vi "Interpolate_Calib_Coeff.vi"(5 "Analysis Info cluster":T1={"Colour"=0, "Inst type"=enum."Pitot-static tube", "Inst name"="Manometer voltage", "Symbol"="U", "Code name"="", "Extra Info"="U", "Inst Array"=enum."PWA", "U"=0.0, "u^2"=0.0, "u^3"=0.0, "u^4"=0.0, "Skew_u"=0.0, "Kurt_u"=0.0, "Sd Error in Mean"=0.0, "% u'/U"=0.0, "X"=0.0, "Y"=0.0, "Z"=0.0, "Timescale integral Estimate"=0.0, "Sd Error in Variance"=0.0, "Calib File"=path "", "Calib Constants"=[], "Output Position"=FALSE, "Stats"=enum."None", "Av Sampling Rate"=0.0, "Av No of Samples"=0.0, "Total Meas Time (s)"=0.0, "OrigChName"="", "Max value"=0.0, "Min value"=0.0, "Req Sample Rate Hz"=0.0, "Sync Delay Time (s)"=0.0, "Ch No"=0, "Device"="", "Use Latest Calib"=FALSE, "Port"="", "Metadata Ch Names"=[], "Metadata Ch Values"=[], "Label"="", "chState"=enum."Solo", "Point Drift"=0.0, "inputConfig"=""} {"Kurt_u" format="%_3g"; "u^4" format="%_3g"; "u^3" format="%_3g"; "Sd Error in Variance" format="%_3g"; "u^2" format="%_3g"; "Sd Error in Mean" format="%_3g"; "U" format="%_3g"; "Sync Delay Time (s)" format="%.4f"; "Total Meas Time (s)" format="%_5g"; "Skew_u" format="%_3g"; "% u'/U" format="%_3g"}, 7 "Take New Data?":bool) -> (0 "Calib Coeff":dbl[](array[numeric]), 1 "Calib Type Name":string, 2 "Calib file string":string, 3 "Read file":bool, 4 "Analysis Info cluster  Out":T1={"Colour"=0, "Inst type"=enum."Pitot-static tube", "Inst name"="Manometer voltage", "Symbol"="U", "Code name"="", "Extra Info"="U", "Inst Array"=enum."PWA", "U"=0.0, "u^2"=0.0, "u^3"=0.0, "u^4"=0.0, "Skew_u"=0.0, "Kurt_u"=0.0, "Sd Error in Mean"=0.0, "% u'/U"=0.0, "X"=0.0, "Y"=0.0, "Z"=0.0, "Timescale integral Estimate"=0.0, "Sd Error in Variance"=0.0, "Calib File"=path "", "Calib Constants"=[], "Output Position"=FALSE, "Stats"=enum."None", "Av Sampling Rate"=0.0, "Av No of Samples"=0.0, "Total Meas Time (s)"=0.0, "OrigChName"="", "Max value"=0.0, "Min value"=0.0, "Req Sample Rate Hz"=0.0, "Sync Delay Time (s)"=0.0, "Ch No"=0, "Device"="", "Use Latest Calib"=FALSE, "Port"="", "Metadata Ch Names"=[], "Metadata Ch Values"=[], "Label"="", "chState"=enum."Solo", "Point Drift"=0.0, "inputConfig"=""} {"Kurt_u" format="%_3g"; "u^4" format="%_3g"; "u^3" format="%_3g"; "Sd Error in Variance" format="%_3g"; "u^2" format="%_3g"; "Sd Error in Mean" format="%_3g"; "U" format="%_3g"; "Sync Delay Time (s)" format="%.4f"; "Total Meas Time (s)" format="%_5g"; "Skew_u" format="%_3g"; "% u'/U" format="%_3g"})   [LabVIEW 2022 SP3]
uses:
  Controls/Inst_type.ctl
  Globals/Meas_global.vi
  <vilib>/Analysis/NI_AALPro.lvlib
  Globals/Plug_in_data_global.vi
  XW calib map/XW_Map_Global.vi
  XW calib map/Map method.ctl
  Globals/Dynamic_call_global.ph.vi
  <vilib>/Analysis/NI_AALBase.lvlib
  <vilib>/Analysis/baseanly.llb/Mean (DBL).vi
  FFID/FFID Calib Constants index.ctl
  CTA/CTA Calib Coeff Global.vi
  Controls/Analysis_info_cluster.ctl
  Controls/Instrument_Array.ctl
  Controls/channelState.ctl
panel:
  out "Volts":dbl
  out "Time":dbl format="%#.0f"
  out "Earlier raw data file":string
  in  "TAKE NEW DATA XW Map method":T5=enum."Const. Psi_eff (std.)"
  in  "Domain padding factor":dbl=1.01
  in  "cap indicial sum to n":bool=TRUE
  in  "surface order (n)":i32=5
  in  "Apply calibration corrections":bool=TRUE
  in  "POST PROC. XW Map method":T5=enum."Psi_eff, k = f(Umagn.)"
  in  "variable n":bool=TRUE
  in  "wire diameter (mu.m)":dbl=5.0
  out "Header info":string[][](array[string])
  # "For polysurface method only:"
  # "For trimesh method only"
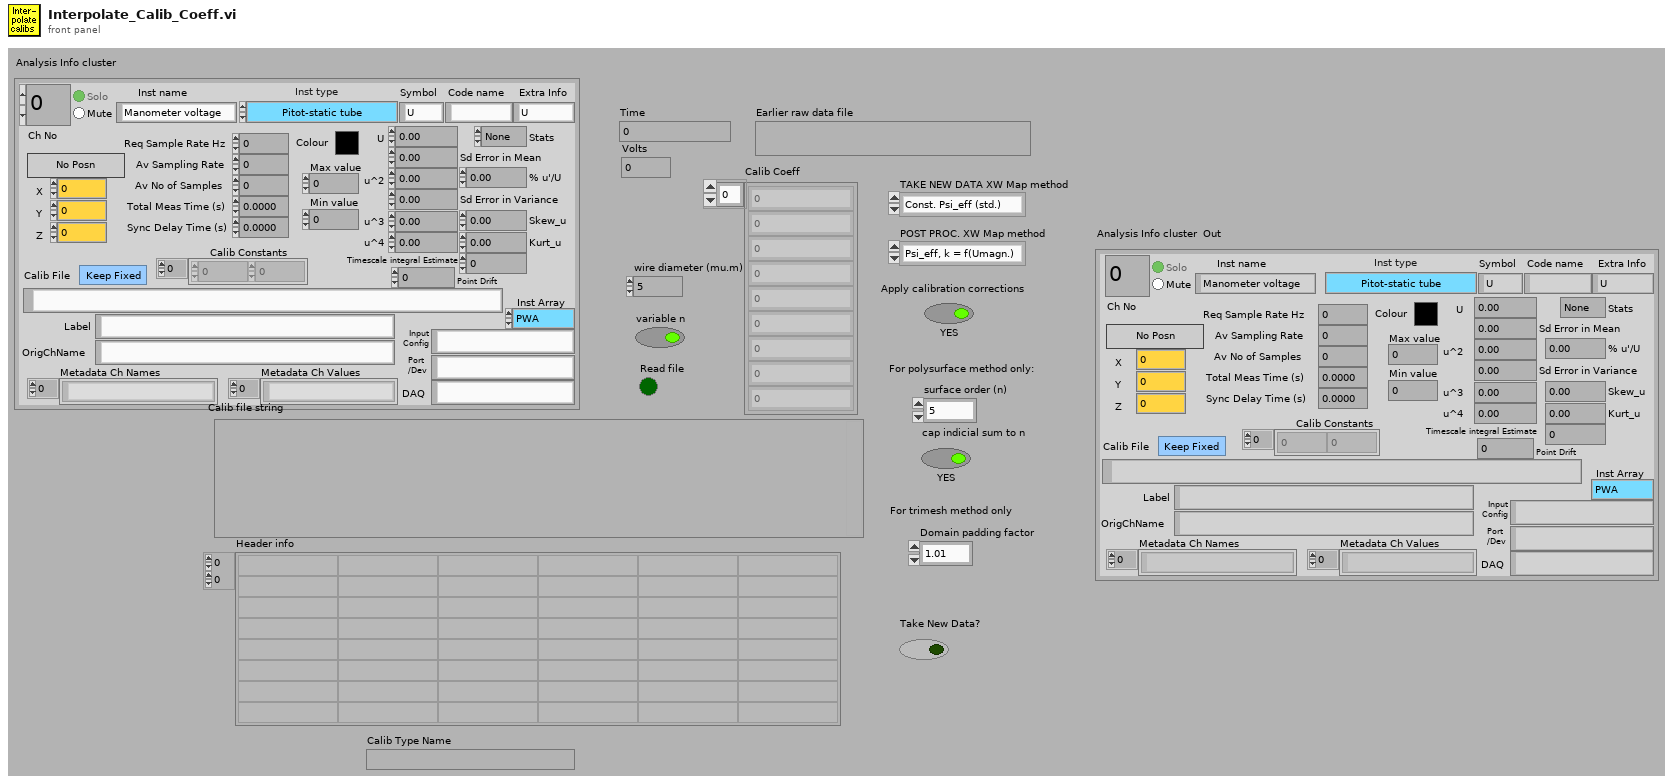
[diagram p1: front panel]
types:
  T1 = typedef "Analysis_info_cluster.ctl" = cluster{"Colour":u32, "Inst type":T2, "Inst name":string, "Symbol":string, "Code name":string, "Extra Info":string, "Inst Array":T3, "U":dbl, "u^2":dbl, "u^3":dbl, "u^4":dbl, "Skew_u":dbl, "Kurt_u":dbl, "Sd Error in Mean":dbl, "% u'/U":dbl, "X":dbl, "Y":dbl, "Z":dbl, "Timescale integral Estimate":dbl, "Sd Error in Variance":dbl, "Calib File":path, "Calib Constants":dbl[], "Output Position":bool, "Stats":enum16{"None", "Basic", "Full"}, "Av Sampling Rate":dbl, "Av No of Samples":dbl, "Total Meas Time (s)":dbl, "OrigChName":string, "Max value":dbl, "Min value":dbl, "Req Sample Rate Hz":dbl, "Sync Delay Time (s)":dbl, "Ch No":i16, "Device":string, "Use Latest Calib":bool, "Port":string, "Metadata Ch Names":string[], "Metadata Ch Values":string[], "Label":string, "chState":T4, "Point Drift":dbl, "inputConfig":string}
  T2 = typedef "Inst_type.ctl" = enum16{"Raw voltage", "Raw with zero offsetting", "Propeller anemometer", "Pressure Transducer", "Pitot-static tube", "Hot wire", "Cross wire 1", "Cross wire 2", "Generic Linear", "Generic Polynomial", "Generic BackPoly", "Fast FID", "Thermocouple", "Cold wire", "Pulsed Wire", "LDA Vel", "LDA Tran time", "LDA Arr time", "Microphone"}
  T3 = typedef "Instrument_Array.ctl" = enum16{"PWA", "LDA", "Analogue"}
  T4 = typedef "channelState.ctl" = enum32{"No Selection", "Solo", "Mute"}
  T5 = typedef "Map method.ctl" = enum16{"Triangle mesh", "Polynomial surface", "Const. Psi_eff (std.)", "Psi_eff = f(Umagn.)", "Psi_eff, k = f(Umagn.)"}
  T6 = cluster{"1st Calib time":dbl, "2nd Calib time":dbl, "Meas start time":dbl, "Meas end time":dbl, "Fraction":dbl}
  T7 = enum16{"Save no data", "Save data in new files", "Save data in existing files"}
  T8 = typedef "Calibration data.ctl" = cluster{"X cal.[]":dbl[], "Re cal.[]":dbl[], "a1[]":dbl[], "a2[]":dbl[], "a3[]":dbl[]}
  T9 = typedef "FFID Calib Constants index.ctl" = u16
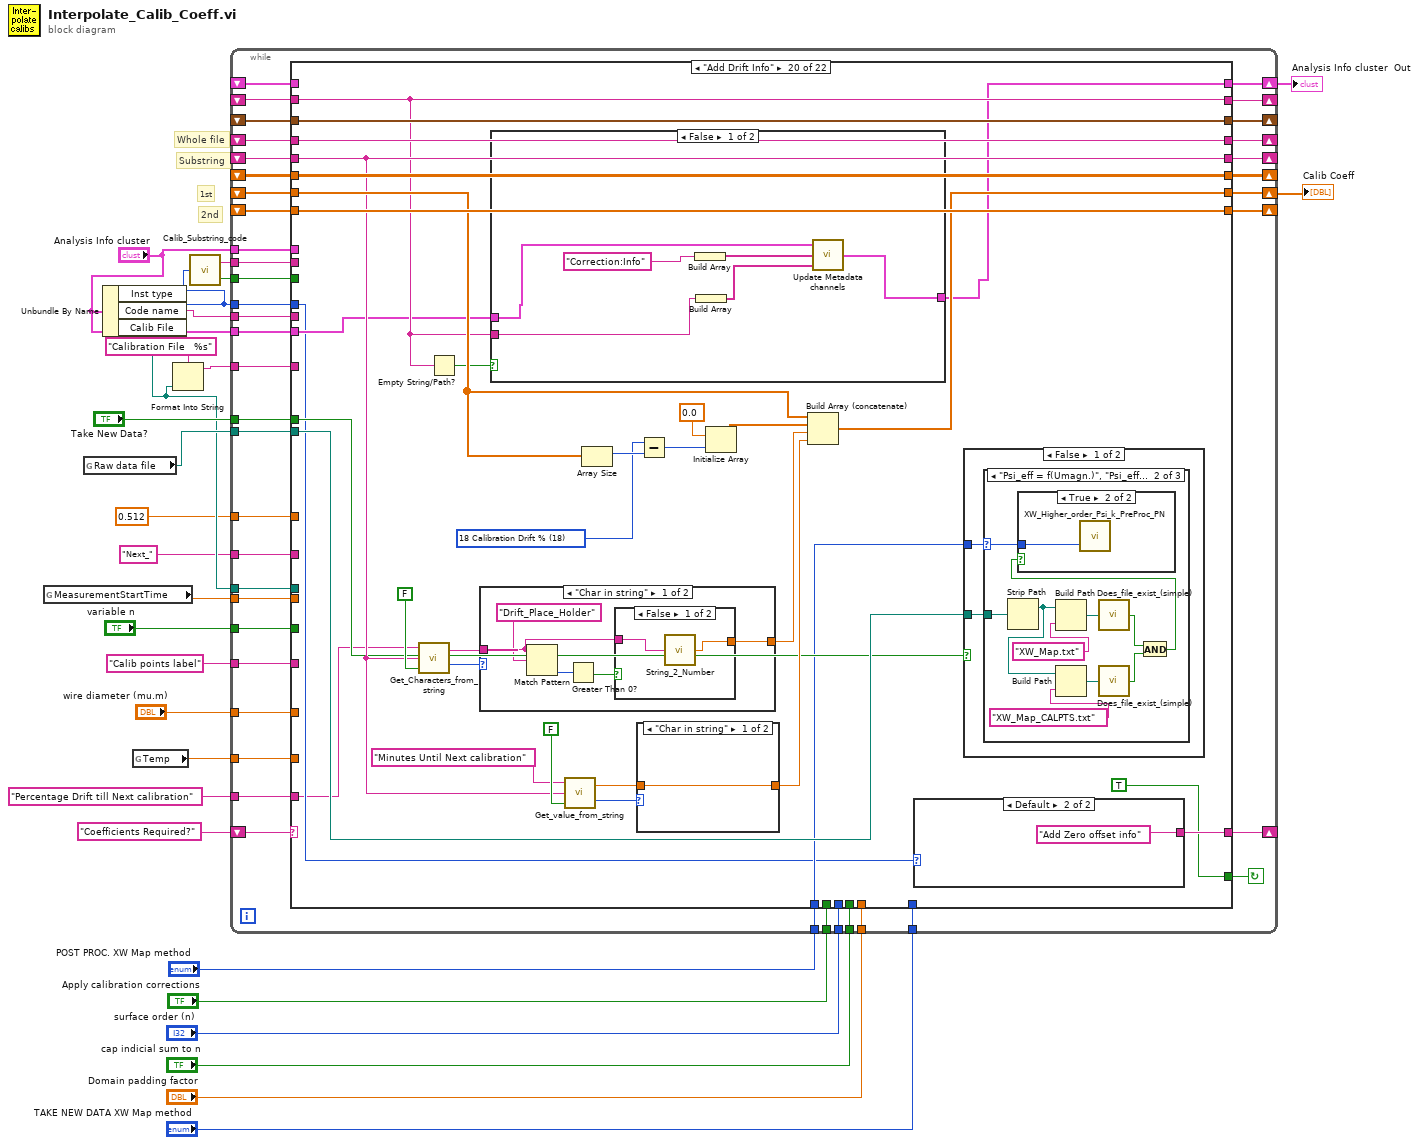
[diagram p0: block diagram]
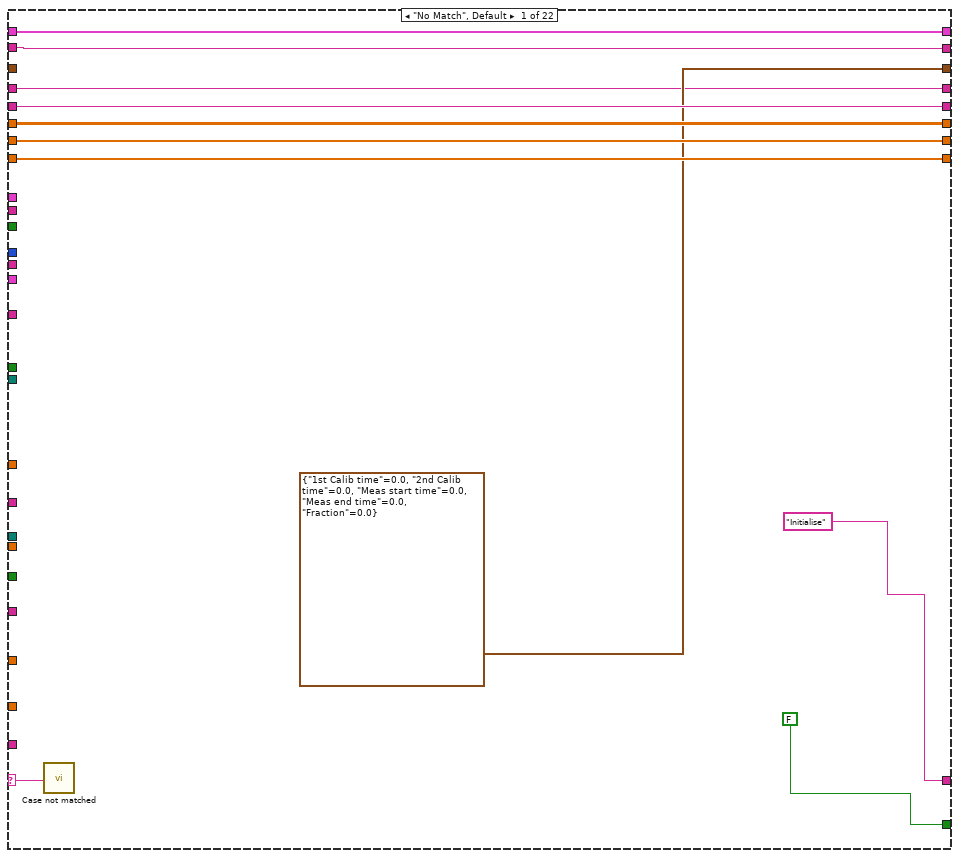
[diagram p2: hidden frame]
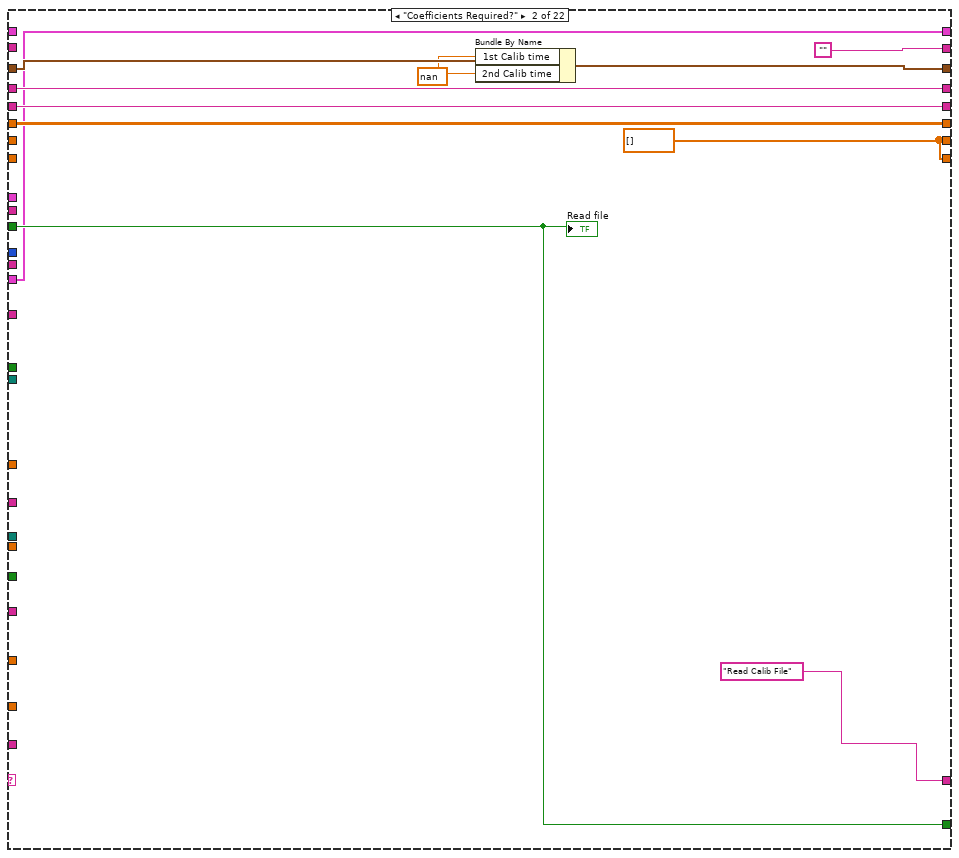
[diagram p3: hidden frame]
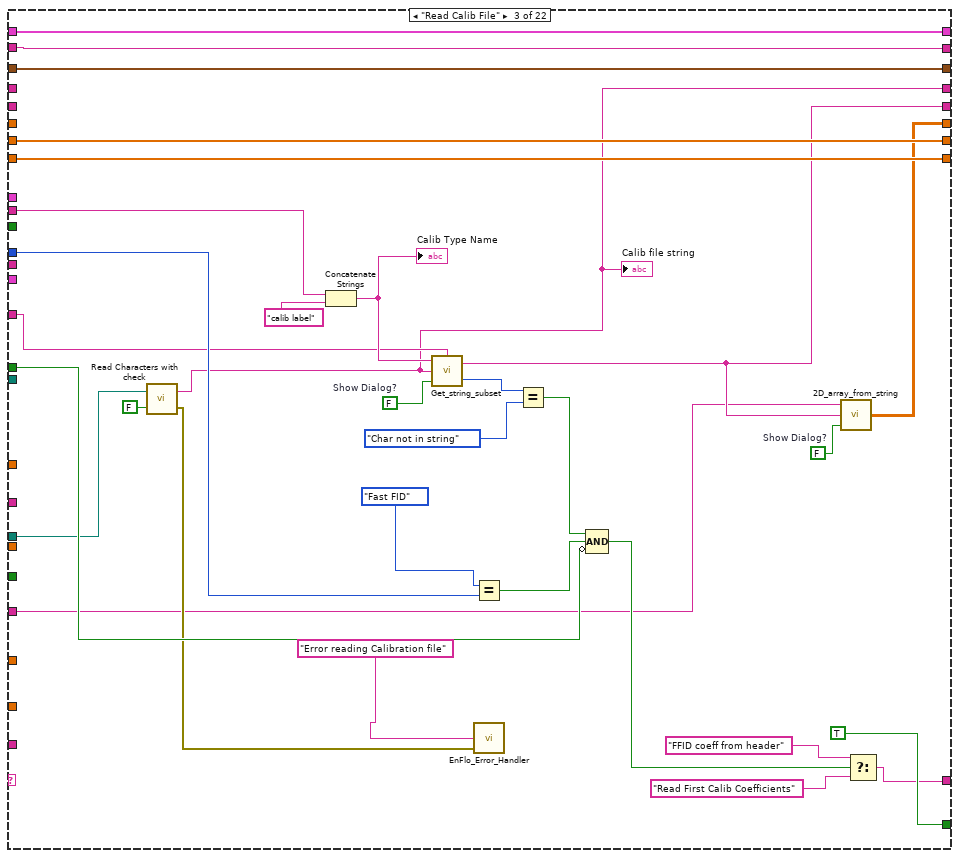
[diagram p4: hidden frame]
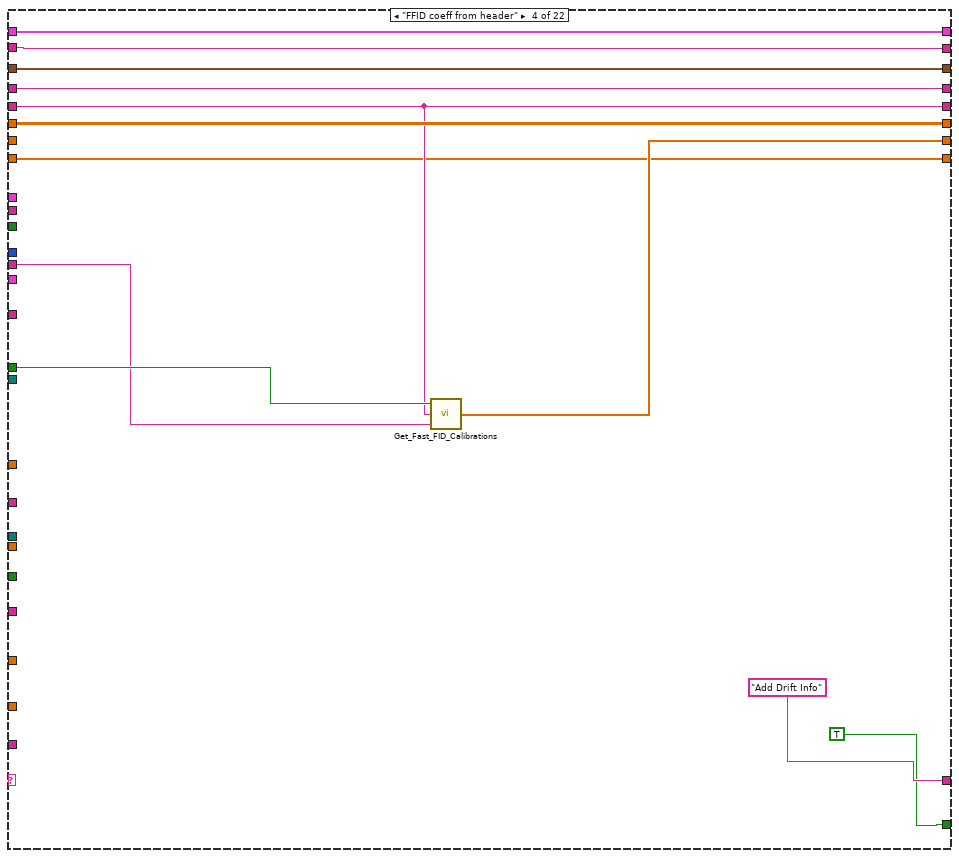
[diagram p5: hidden frame]
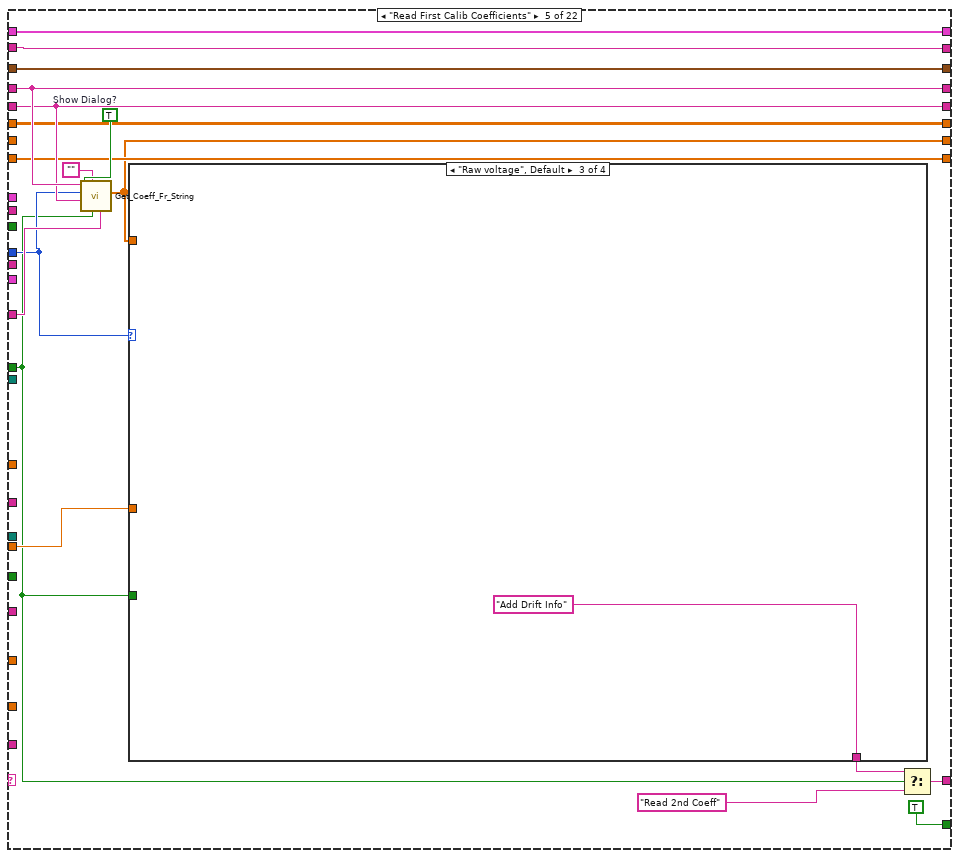
[diagram p6: hidden frame]
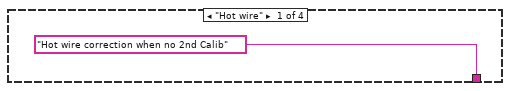
[diagram p7: hidden frame]
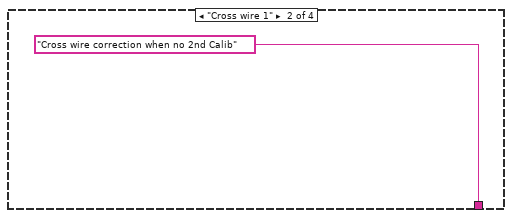
[diagram p8: hidden frame]
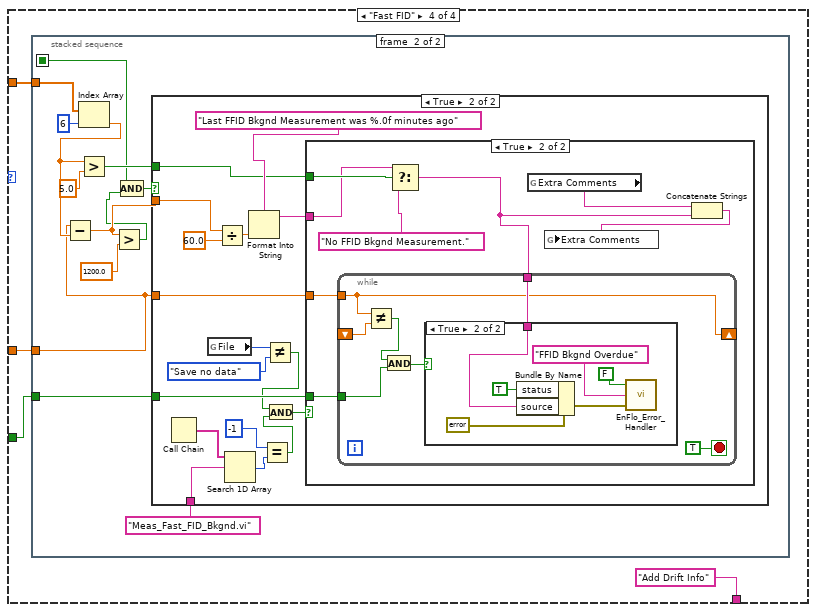
[diagram p9: hidden frame]
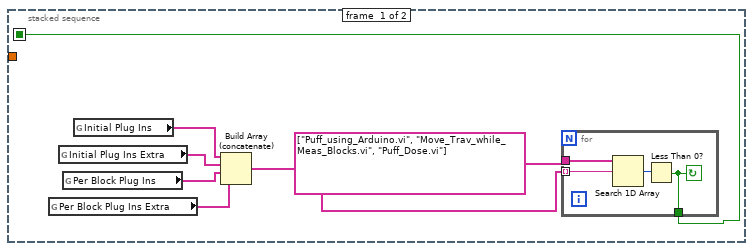
[diagram p10: hidden frame]
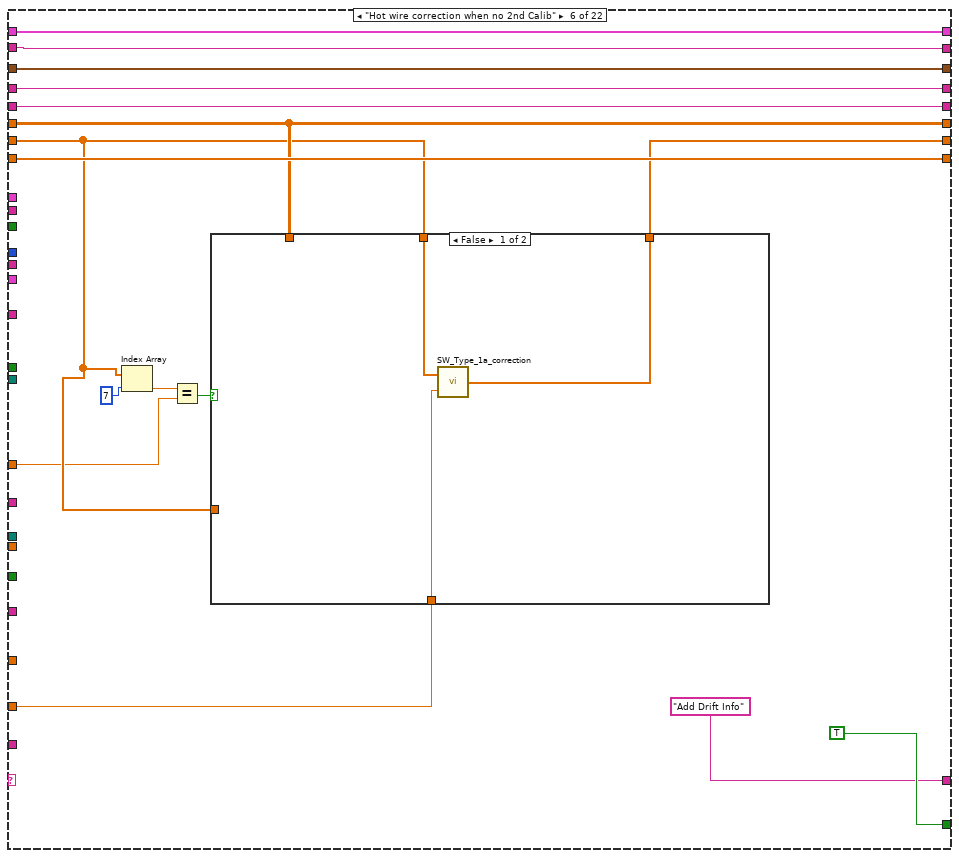
[diagram p14: hidden frame]
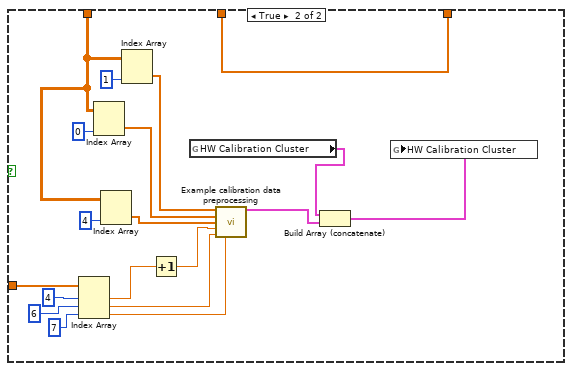
[diagram p15: hidden frame]
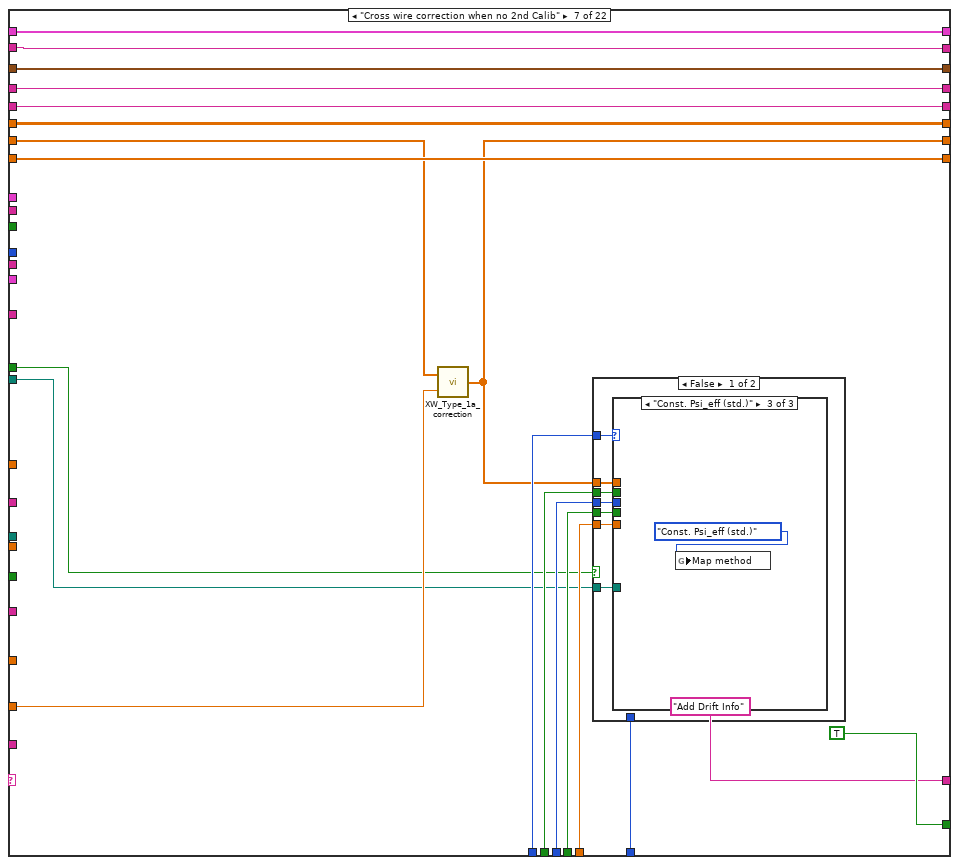
[diagram p16: hidden frame]
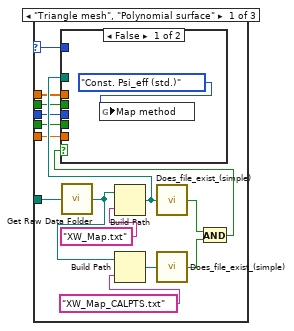
[diagram p17: hidden frame]
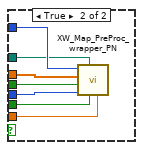
[diagram p18: hidden frame]
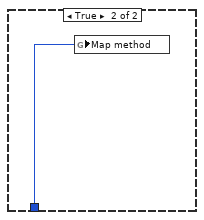
[diagram p20: hidden frame]
diagram:
  # "Substring"
  # "2nd"
  # "Whole file"
  # "1st"
  n1 = global read "Meas_global.vi" "MeasurementStartTime"() -> (w5:dbl)
  n2 = global read "Meas_global.vi" "Raw data file"() -> (w21:path)
  n3 = Unbundle By Name("Analysis Info cluster") -> ("Inst type"=w24:T2, "Code name"=w25:string, "Calib File"=w7:path)
  n4 = global read "Meas_global.vi" "Temp"() -> (w20:dbl)
  n5 = Format Into String(format string="Calibration File   %s", w7) -> (resulting string=w8:string)  [unwired: 2 in, 1 out]
  n6 = call "Calib_Substring_code.vi"("Inst type"=w24) -> ("Substring Type"=w22:string, "Read file"=w23:bool)
  n7 = while {
    tunnel: w7 -> [w61]
    shift-left: _ -> [w62]
    shift-right: [w63] -> _
    shift-left: _ -> [w64]
    shift-right: [w66] -> w27
    tunnel: w24 -> [w68]
    shift-left: _ -> [w65]
    shift-right: [w67] -> _
    shift-left: "Coefficients Required?" -> [w69]
    shift-right: [w34] -> _
    tunnel: "Take New Data?" -> [w60]
    tunnel: w25 -> [w59]
    shift-right: [w58] -> _
    shift-left: _ -> [w57]
    shift-right: [w56] -> _
    shift-left: _ -> [w55]
    shift-right: [w54] -> _
    shift-left: _ -> [w53]
    tunnel: w23 -> [w52]
    tunnel: w22 -> [w51]
    tunnel: w21 -> [w50]
    shift-right: [w49] -> _
    shift-left: _ -> [w48]
    tunnel: w20 -> [w47]
    tunnel: "wire diameter (mu.m)" -> [w46]
    tunnel: "variable n" -> [w45]
    tunnel: "POST PROC. XW Map method" -> [w44]
    tunnel: "Apply calibration corrections" -> [w43]
    tunnel: "surface order (n)" -> [w42]
    tunnel: "cap indicial sum to n" -> [w41]
    tunnel: "Domain padding factor" -> [w40]
    tunnel: "TAKE NEW DATA XW Map method" -> [w39]
    tunnel: "Analysis Info cluster" -> [w38]
    shift-right: [w36] -> w11
    shift-left: _ -> [w37]
    tunnel: "Analysis Info cluster" -> [w35]
    tunnel: w8 -> [w33]
    tunnel: w5 -> [w32]
    tunnel: 0.512 ("y") -> [w31]
    tunnel: "Next_" -> [w30]
    tunnel: "Calib points label" -> [w29]
    tunnel: "Percentage Drift till Next calibration" ("Variable name") -> [w28]
    stop <- w70 continue-if-true
    n8 = case shown="\"Add Drift Info\"" w69 {
      selector: w69 -> [w71 _ _ _ _ _ _ _ _ _ _ _ _ _ _ _ _ _ _ _ _ _]
      tunnel: [FALSE w87 TRUE ("Read file") TRUE TRUE ("Read file") TRUE ("Read file") TRUE ("Read file") TRUE ("Read file") TRUE ("Read file") TRUE ("Read file") TRUE ("Read file") TRUE ("Read file") TRUE ("Read file") TRUE ("Read file") TRUE ("Read file") TRUE ("Read file") w744 w1170 TRUE ("Read file") TRUE ("Read file") TRUE ("Read file") FALSE ("Read file")] -> w70
      tunnel: ["Initialise" "Read Calib File" w111 "Add Drift Info" w143 "Add Drift Info" "Add Drift Info" w325 w375 w396 w410 w446 "Bkgnd info from header" ("f") "Add Drift Info" ("f") "Add Drift Info" ("f") "Add Drift Info" ("f") w745 w1171 "Add Drift Info" w1316 "Add Zero offset info" ("f") "End" ("f")] -> w34
      tunnel: w68 -> [_ _ w118 _ w139 _ _ w321 _ _ _ w432 _ _ _ _ _ _ _ w1290 _ w1383]
      tunnel: [w79 w91 w95 w131 w151 w237 w279 w315 w369 w390 w424 w449 w490 w521 w537 w697 w752 w1178 w1265 w1302 w1370 w1388] -> w67
      tunnel: [w78 w89 w108 w129 w136 w231 w262 w316 w374 w395 w425 w448 w463 w497 w540 w657 w748 w1174 w1257 w1296 w1355 w1379] -> w66
      tunnel: w65 -> [w79 w91 _ w131 w151 w237 w279 w315 w369 w390 w424 w449 w490 w521 w543 w697 w753 w1179 w1265 w1302 w1370 w1388]
      tunnel: w64 -> [w78 _ w108 _ _ w225 w270 w316 w374 w395 w425 w448 w462 w499 w541 w681 w749 w1175 w1258 w1310 w1363 w1378]
      tunnel: [w77 w90 w94 w135 w150 w228 w278 w328 w377 w398 w427 w428 w479 w515 w542 w671 w751 w1177 w1261 w1318 w1364 w1387] -> w63
      tunnel: w62 -> [w77 w90 _ w135 w150 w228 w278 w328 w377 w398 w427 w428 w479 w515 w542 w671 w750 w1176 w1261 w1318 w1364 w1387]
      tunnel: w61 -> [_ _ w100 _ _ _ _ _ _ _ _ _ _ _ _ _ _ _ _ _ _ w1385]
      tunnel: w60 -> [_ _ w114 w132 w137 _ w265 w326 _ _ _ _ _ _ _ w659 _ _ _ w1294 _ _]
      tunnel: w59 -> [_ _ _ w130 _ _ _ _ _ _ _ _ _ _ _ _ w756 w1182 _ _ _ _]
      tunnel: [w76 w89 w107 w128 w149 w236 w277 w317 w361 w382 w422 w433 w483 w501 w558 w682 w747 w1173 w1264 w1317 w1369 w1386] -> w58
      tunnel: w57 -> [w76 _ w107 w128 w149 w236 w277 _ w361 w382 w422 w433 w483 w501 w558 w682 w746 w1172 w1264 w1317 w1369 w1386]
      tunnel: [w74 w88 w99 w126 w152 w238 w280 w329 w378 w381 w421 w445 w480 w516 w567 w694 w754 w1180 w1262 w1319 w1371 w1389] -> w56
      tunnel: w55 -> [w74 w88 _ w126 w152 w238 w280 w329 w378 _ w421 w445 w480 w516 w567 w694 w757 w1183 w1262 w1319 w1371 w1389]
      tunnel: [T6 {"1st Calib time"=0.0, "2nd Calib time"=0.0, "Meas start time"=0.0, "Meas end time"=0.0, "Fraction"=0.0} w85 w106 w127 w147 w234 w275 w314 w365 w386 w423 w434 w481 w517 w568 w695 w743 w1169 w1263 w1299 w1372 w1390] -> w54
      tunnel: w53 -> [_ w86 w106 w127 w147 w234 w275 w314 w368 w389 w420 w436 w481 w517 w568 w695 w755 w1181 w1263 w1299 w1372 w1390]
      tunnel: w52 -> [_ w87 _ _ _ _ _ _ _ _ _ _ _ _ _ _ _ _ _ _ _ _]
      tunnel: w51 -> [_ _ w105 _ _ _ _ _ _ _ _ _ _ _ _ _ _ _ _ _ _ _]
      tunnel: w50 -> [_ _ _ _ _ _ w264 _ _ _ w408 _ _ _ _ w660 w739 _ _ w1295 _ _]
      tunnel: [w73 "" w104 w125 w145 w233 w274 w322 w360 w380 w409 w430 w470 w506 w559 w686 w742 w1167 w1255 w1298 w1373 w1391] -> w49
      tunnel: w48 -> [w73 _ w104 w125 w145 w233 w274 w322 w360 w380 w409 w430 w472 w508 w561 w688 w741 w1168 w1256 w1298 w1373 w1391]
      tunnel: w47 -> [_ _ _ _ _ w230 w272 _ _ _ _ _ _ _ w552 w662 _ _ _ _ _ _]
      tunnel: w46 -> [_ _ _ _ _ _ _ _ _ _ _ _ _ _ w550 w661 _ _ _ _ _ _]
      tunnel: w45 -> [_ _ _ _ _ _ _ _ _ _ _ _ _ _ w551 w663 _ _ _ _ _ _]
      tunnel: w44 -> [_ _ _ _ _ _ w271 _ _ _ _ _ _ _ _ w658 _ _ _ w1293 _ _]
      tunnel: w43 -> [_ _ _ _ _ _ w269 _ _ _ _ _ _ _ _ w656 _ _ _ _ _ _]
      tunnel: w42 -> [_ _ _ _ _ _ w268 _ _ _ _ _ _ _ _ w655 _ _ _ _ _ _]
      tunnel: w41 -> [_ _ _ _ _ _ w267 _ _ _ _ _ _ _ _ w654 _ _ _ _ _ _]
      tunnel: w40 -> [_ _ _ _ _ _ w266 _ _ _ _ _ _ _ _ w653 _ _ _ _ _ _]
      tunnel: w39 -> [_ _ _ _ _ _ w263 _ _ _ _ _ _ _ _ _ _ _ _ _ _ _]
      tunnel: w38 -> [_ w83 _ _ _ _ _ _ _ _ _ _ _ _ _ _ _ _ _ w1292 _ _]
      tunnel: w37 -> [w72 _ w102 w124 w142 w229 w261 w319 w359 w379 w405 w429 w469 w505 w549 w652 w740 w1166 w1254 _ w1374 w1392]
      tunnel: [w72 w83 w102 w124 w142 w229 w261 w319 w359 w379 w405 w429 w469 w505 w549 w652 w740 w1166 w1254 w1291 w1374 w1392] -> w36
      tunnel: w35 -> [_ _ _ _ _ _ _ _ _ _ _ _ _ _ _ _ _ _ _ _ _ _]
      tunnel: w33 -> [_ _ w101 _ w141 _ _ w318 _ _ _ _ _ _ _ _ _ _ _ _ _ _]
      tunnel: w32 -> [_ _ _ _ w138 _ _ _ _ _ _ _ _ _ _ _ _ w1165 _ _ _ w1375]
      tunnel: w31 -> [_ _ _ _ _ w223 _ _ _ _ _ _ _ _ w546 _ _ _ _ _ _ _]
      tunnel: w30 -> [_ _ _ _ _ _ _ w313 _ _ _ _ _ _ w539 _ _ _ _ _ _ _]
      tunnel: w29 -> [_ _ w93 _ _ _ _ _ _ _ _ _ _ _ w544 _ _ _ _ _ _ _]
      tunnel: w28 -> [_ _ _ _ _ _ _ _ _ _ _ _ _ _ w538 _ _ _ _ w1288 _ _]
      frame "No Match", Default {
        n9 = call "Case not matched.vi"("Case Name not Matched"=w71) -> ()
      }
      frame "Coefficients Required?" {
        w82 = nan ("1st Calib time")
        w89 = dbl[] [] ("Calib Coeff")
        n10 = Bundle By Name(cluster=w86, "1st Calib time"=w82, "2nd Calib time"=w82) -> (w85:T6)
        "Read file" <- w87
      }
      frame "Read Calib File" {
        w96 = FALSE  # Show Dialog?
        w119 = FALSE  # Show Dialog?
        n11 = call "Read Characters with check.vi"("Call EnFlo Error Handler?"=FALSE, "file (use dialog)"=w100) -> ("error out"=w98:errorcluster, "Read String"=w99:string)
        "Calib file string" <- w99
        n12 = Concatenate Strings(w105, "calib label") -> (w122:string)
        "Calib Type Name" <- w122
        n13 = call "Get_string_subset.vi"("String Name"=w101, "Show Dialog?"=w119, "String to split"=w99, "File Label"=w122) -> ("Status"=w121:enum16{"Char in string", "Char not in string"}, "Output string"=w95:string)
        n14 = Equal?(x=Inst_type."Fast FID" ("Inst type"), y=w118) -> (x = y?=w115:bool)
        n15 = call "EnFlo_Error_Handler.vi"("error in (no error)"=w98, "Error Type"="Error reading Calibration file") -> ()  [unwired: 1 in, 3 out]
        n16 = Equal?(x=w121, y=enum16{"Char in string", "Char not in string"}."Char not in string" ("Status")) -> (x = y?=w116:bool)
        n17 = Compound Arithmetic op=AND(w116, w115, invert w114) -> (w112:bool)
        n18 = call "2D_array_from_string.vi"("Show Dialog?"=w96, "Input string"=w95, "Array title"=w93) -> ("2D data array"=w94:dbl[][])  [unwired: 1 in]
        n19 = Select(t="FFID coeff from header", s=w112, f="Read First Calib Coefficients") -> (s? t:f=w111:string)
      }
      frame "FFID coeff from header" {
        n20 = call "Get_Fast_FID_Calibrations.vi"("Code Name"=w130, "Calib File String"=w131, "Take New Data"=w132) -> ("Calib Constants"=w129:dbl[])
      }
      frame "Read First Calib Coefficients" {
        w153 = TRUE  # Show Dialog?
        n21 = call "Get_Coeff_Fr_String.vi"("String Name"=w141, "Take New Data?"=w137, "Prefix"="", "Show Dialog?"=w153, "Sub String"=w151, "Inst type"=w139, "Whole String"=w152) -> ("Calib Constants"=w136:dbl[])  [unwired: 2 in, 1 out]
        n22 = case shown="\"Raw voltage\", Default" w139 {
          tunnel: ["Hot wire correction when no 2nd Calib" "Cross wire correction when no 2nd Calib" "Add Drift Info" "Add Drift Info"] -> w144
          tunnel: w138 -> [_ _ _ w158]
          tunnel: w137 -> [_ _ _ w159]
          tunnel: w136 -> [_ _ _ w157]
          frame "Hot wire" {
          }
          frame "Cross wire 1" {
          }
          frame "Raw voltage", Default {
          }
          frame "Fast FID" {
            n23 = stacked-sequence {
              seq-local: [w161 _] -> [_ w172]
              tunnel: w159 -> [_ w181]
              tunnel: w158 -> [_ w174]
              tunnel: w157 -> [_ w173]
              frame #0 {
                n24 = global read "Dynamic_call_global.ph.vi" "Per Block Plug Ins Extra"() -> (w164:string[])
                n25 = global read "Dynamic_call_global.ph.vi" "Initial Plug Ins Extra"() -> (w166:string[])
                n26 = global read "Dynamic_call_global.ph.vi" "Per Block Plug Ins"() -> (w165:string[])
                n27 = global read "Dynamic_call_global.ph.vi" "Initial Plug Ins"() -> (w167:string[])
                n28 = Build Array (concatenate)(w167, w166, w165, w164) -> (w163:string[])
                n29 = for {
                  tunnel: string[] ["Puff_using_Arduino.vi", "Move_Trav_while_Meas_Blocks.vi", "Puff_Dose.vi"] ("appended array") -> [w171]
                  tunnel: w163 -> [w170] mode=indexing
                  tunnel: [w168] -> w161
                  stop <- w168 continue-if-true
                  n30 = Search 1D Array(1D array=w171, element=w170) -> (index of element=w169:i32)  [unwired: 1 in]
                  n31 = Less Than 0?(x=w169) -> (x < 0?=w168:bool)
                }
              }
              frame #1 {
                n32 = Index Array(array=w173, index=6) -> (element=w180:dbl)
                n33 = Subtract(x=w174, y=w180) -> (x-y=w182:dbl)
                n34 = Greater?(x=w180, y=5.0) -> (0:w177:bool)
                n35 = Greater?(x=w182, y=1200.0) -> (0:w176:bool)
                n36 = Compound Arithmetic op=AND(w172, w176) -> (w175:bool)
                n37 = case shown="True" w175 {
                  tunnel: w182 -> [_ w201]
                  tunnel: w181 -> [_ w200]
                  tunnel: "Meas_Fast_FID_Bkgnd.vi" -> [_ w198]
                  tunnel: w177 -> [_ w194]
                  tunnel: w174 -> [_ w185]
                  frame False {
                  }
                  frame True {
                    n38 = Call Chain() -> (call chain=w199:string[])
                    n39 = global read "Meas_global.vi" "File"() -> (w191:T7)
                    n40 = Divide(x=w201, y=60.0) -> (x/y=w197:dbl)
                    n41 = Search 1D Array(1D array=w199, element=w198) -> (index of element=w190:i32)  [unwired: 1 in]
                    n42 = Format Into String(format string="Last FFID Bkgnd Measurement was %.0f minutes ago", w197) -> (resulting string=w193:string)  [unwired: 2 in, 1 out]
                    n43 = Equal?(x=-1, y=w190) -> (x = y?=w188:bool)
                    n44 = Not Equal?(x=w191, y=T7."Save no data" ("File")) -> (x != y?=w187:bool)
                    n45 = And(x=w187, y=w188) -> (x .and. y?=w186:bool)
                    n46 = case shown="True" w186 {
                      tunnel: w200 -> [_ w209]
                      tunnel: w194 -> [_ w206]
                      tunnel: w193 -> [_ w205]
                      tunnel: w185 -> [_ w202]
                      frame False {
                      }
                      frame True {
                        n47 = Select(t=w205, s=w206, f="No FFID Bkgnd Measurement.") -> (s? t:f=w203:string)
                        n48 = while {
                          tunnel: w209 -> [w212]
                          tunnel: w203 -> [w216]
                          shift-right: [w214] -> _
                          shift-left: _ -> [w215]
                          tunnel: w202 -> [w214]
                          stop <- TRUE stop-if-true
                          n49 = Not Equal?(x=w214, y=w215) -> (x != y?=w213:bool)
                          n50 = And(x=w213, y=w212) -> (x .and. y?=w211:bool)
                          n51 = case shown="True" w211 {
                            tunnel: w216 -> [_ w220]
                            frame False {
                            }
                            frame True {
                              n52 = Bundle By Name(cluster=errorcluster {"status"=FALSE, "code"=0, "source"=""} ("error in (no error)"), "status"=TRUE, "source"=w220) -> (w219:errorcluster)
                              n53 = call "EnFlo_Error_Handler.vi"("error in (no error)"=w219, "Error Type"="FFID Bkgnd Overdue", "Dialog Box (F)"=FALSE ("Dialog Box (T)")) -> ()  [unwired: 1 in, 2 out]
                            }
                          }
                        }
                        n54 = global read "Meas_global.vi" "Extra Comments"() -> (w208:string)
                        n55 = Concatenate Strings(w208, w203) -> (w207:string)
                        n56 = global write "Meas_global.vi" "Extra Comments"(w207) -> ()
                      }
                    }
                  }
                }
              }
            }
          }
        }
        n57 = Select(t=w144, s=w137, f="Read 2nd Coeff") -> (s? t:f=w143:string)
      }
      frame "Hot wire correction when no 2nd Calib" {
        n58 = Index Array(array=w225, index=7) -> (element=w226:dbl)
        n59 = Equal?(x=w226, y=w223) -> (x = y?=w224:bool)
        n60 = case shown="False" w224 {
          tunnel: w225 -> [w241 w260]
          tunnel: [w240 w260] -> w231
          tunnel: w230 -> [w239 _]
          tunnel: w228 -> [_ w254]
          tunnel: w225 -> [_ w252]
          frame False {
            n61 = call "SW_Type_1a_correction.vi"("Tmeas (degC)"=w239, "Calib consts."=w241) -> ("Corrected calib consts."=w240:dbl[])
          }
          frame True {
            n62 = Index Array(array=w252, index #1=4 ("index"), index #2=6 ("index"), index #3=7 ("index")) -> (element #1=w250:dbl, element #2=w249:dbl, element #3=w248:dbl)
            n63 = Index Array(array=w254, index (col)=0 ("disabled index (col)")) -> (element=w258:dbl[])  [unwired: 1 in]
            n64 = Index Array(array=w254, index (col)=4 ("disabled index (col)")) -> (element=w253:dbl[])  [unwired: 1 in]
            n65 = Index Array(array=w254, index (col)=1 ("disabled index (col)")) -> (element=w256:dbl[])  [unwired: 1 in]
            n66 = Increment(x=w250) -> (x+1=w242:dbl)
            n67 = global read "CTA Calib Coeff Global.vi" "HW Calibration Cluster"() -> (w245:T8[])
            n68 = call "Example calibration data preprocessing.vi"("Vout_cal (V)"=w256, "U_cal (m/s)"=w258, "Ta_cal (°C)"=w253, "Overheat ratio"=w242, "Gain"=w249, "Offset (V)"=w248) -> ("Calibration data"=w244:T8)  [unwired: 9 in]
            n69 = Build Array (concatenate)(w245, w244) -> (w243:T8[])
            n70 = global write "CTA Calib Coeff Global.vi" "HW Calibration Cluster"(w243) -> ()
          }
        }
      }
      frame "Cross wire correction when no 2nd Calib" {
        n71 = call "XW_Type_1a_correction.vi"("Tmeas (degC)"=w272, "Calib consts."=w270) -> ("Corrected calib consts."=w262:dbl[])
        n72 = case shown="False" w265 {
          tunnel: w264 -> [w287 _]
          tunnel: w271 -> [w281 _]
          tunnel: w262 -> [w286 _]
          tunnel: w269 -> [w285 _]
          tunnel: w268 -> [w284 _]
          tunnel: w267 -> [w283 _]
          tunnel: w266 -> [w282 _]
          tunnel: w263 -> [_ w312]
          frame False {
            n73 = case shown="\"Const. Psi_eff (std.)\"" w281 {
              selector: w281 -> [w295 _ _]
              tunnel: w287 -> [w289 _ _]
              tunnel: w286 -> [w300 _ _]
              tunnel: w285 -> [w299 _ _]
              tunnel: w284 -> [w298 _ _]
              tunnel: w283 -> [w297 _ _]
              tunnel: w282 -> [w296 _ _]
              frame "Triangle mesh", "Polynomial surface" {
                n74 = call "Get Raw Data Folder.vi"("Raw data file"=w289) -> ("Main Raw Data Folder"=w288:path)
                n75 = Build Path(base path=w288, name or relative path="XW_Map.txt") -> (appended path=w301:path)
                n76 = Build Path(base path=w288, name or relative path="XW_Map_CALPTS.txt") -> (appended path=w294:path)
                n77 = call "Does_file_exist_(simple).vi"("Pathname"=w301) -> ("exists?"=w291:bool)
                n78 = call "Does_file_exist_(simple).vi"("Pathname"=w294) -> ("exists?"=w292:bool)
                n79 = And(x=w291, y=w292) -> (x .and. y?=w290:bool)
                n80 = case shown="False" w290 {
                  tunnel: w301 -> [_ w309]
                  tunnel: w295 -> [_ w310]
                  tunnel: w300 -> [_ w308]
                  tunnel: w299 -> [_ w307]
                  tunnel: w298 -> [_ w306]
                  tunnel: w297 -> [_ w305]
                  tunnel: w296 -> [_ w304]
                  frame False {
                    n81 = global write "XW_Map_Global.vi" "Map method"(Map_method."Const. Psi_eff (std.)" ("Map method")) -> ()
                  }
                  frame True {
                    n82 = call "XW_Map_PreProc_wrapper_PN.vi"("Domain padding factor"=w304, "cap indicial sum to n"=w305, "XW_Calib_Map file path"=w309, "surface order (n)"=w306, "Apply calibration corrections"=w307, "Calib const"=w308, "Map method"=w310) -> ()  [unwired: 5 out]
                  }
                }
              }
              frame "Psi_eff = f(Umagn.)", "Psi_eff, k = f(Umagn.)" {
              }
              frame "Const. Psi_eff (std.)" {
                n83 = global write "XW_Map_Global.vi" "Map method"(Map_method."Const. Psi_eff (std.)" ("Map method")) -> ()
              }
            }
          }
          frame True {
            n84 = global write "XW_Map_Global.vi" "Map method"(w312) -> ()
          }
        }
      }
      frame "Read 2nd Coeff" {
        (unwired) "Next_Seconds since 1/1/04" ("Variable name")
        w330 = FALSE  # Show Dialog?
        n85 = Equal?(x=w321, y=Inst_type."Fast FID" ("Inst type")) -> (x = y?=w323:bool)
        n86 = call "Get_Coeff_Fr_String.vi"("String Name"=w318, "Take New Data?"=w326, "Prefix"=w313, "Show Dialog?"=w330, "Sub String"=w315, "Inst type"=w321, "Whole String"=w329) -> ("Coefficients Found?"=w320:bool, "Calib Constants"=w317:dbl[])  [unwired: 2 in]
        n87 = case shown="False" w323 {
          tunnel: [w332 w342] -> w325
          tunnel: w320 -> [w334 w343]
          tunnel: w321 -> [w335 _]
          tunnel: w317 -> [_ w340]
          tunnel: w316 -> [_ w339]
          frame False {
            n88 = case shown="\"Raw voltage\", Default" w335 {
              tunnel: ["Hot wire correction when no 2nd Calib" "Cross wire correction when no 2nd Calib" "Add Drift Info"] -> w333
              frame "Hot wire" {
              }
              frame "Cross wire 1" {
              }
              frame "Raw voltage", Default {
              }
            }
            n89 = Select(t="Get Calibration times", s=w334, f=w333) -> (s? t:f=w332:string)
          }
          frame True {
            n90 = case shown="True" w343 {
              tunnel: [w344 w346] -> w342
              tunnel: "Get Measurement times" -> [w344 w347]
              tunnel: w340 -> [_ w357]
              tunnel: w339 -> [_ w355]
              frame False {
              }
              frame True {
                n91 = Index Array(array=w357, index=1) -> (element=w354:dbl)
                n92 = Index Array(array=w355, index=1) -> (element=w353:dbl)
                n93 = Absolute Value(x=w354) -> (abs(x)=w352:dbl)
                n94 = Absolute Value(x=w353) -> (abs(x)=w351:dbl)
                n95 = Divide(x=w352, y=w351) -> (x/y=w350:dbl)
                n96 = Less?(x=w350, y=30.0) -> (x < y?=w345:bool)
                n97 = Select(t="Get Calibration times", s=w345, f=w347) -> (s? t:f=w346:string)
              }
            }
          }
        }
      }
      frame "Get Calibration times" {
        n98 = call "Get_value_from_string.vi"("Input string"=w369, "Variable name"="Seconds since 1/1/04") -> ("Value"=w367:dbl)  [unwired: 1 in, 1 out]
        n99 = call "Get_value_from_string.vi"("Input string"=w369, "Variable name"="Next_Seconds since 1/1/04") -> ("Status"=w364:enum16{"Char in string", "Char not in string"}, "Value"=w366:dbl)  [unwired: 1 in]
        n100 = Equal?(x=w364, y=enum16{"Char in string", "Char not in string"}."Char in string" ("Status")) -> (x = y?=w362:bool)
        n101 = Bundle By Name(cluster=w368, "1st Calib time"=w367, "2nd Calib time"=w366) -> (w365:T6)
        n102 = Select(t="Get Measurement times", s=w362, f="Add Drift Info") -> (s? t:f=w375:string)
      }
      frame "Get Measurement times" {
        n103 = global read "Meas_global.vi" "Pre Setup String"() -> (w381:string)
        n104 = call "Get_value_from_string.vi"("Input string"=w381, "Variable name"="Seconds since 1/1/04") -> ("Value"=w388:dbl)  [unwired: 1 in, 1 out]
        n105 = call "Get_value_from_string.vi"("Input string"=w381, "Variable name"="Measurement_End_Time_Seconds") -> ("Status"=w385:enum16{"Char in string", "Char not in string"}, "Value"=w387:dbl)  [unwired: 1 in]
        n106 = Equal?(x=w385, y=enum16{"Char in string", "Char not in string"}."Char in string" ("Status")) -> (x = y?=w383:bool)
        n107 = Bundle By Name(cluster=w389, "Meas start time"=w388, "Meas end time"=w387) -> (w386:T6)
        n108 = Select(t="Get Calib Points array", s=w383, f="Estimate End time") -> (s? t:f=w396:string)
      }
      frame "Estimate End time" {
        n109 = Unbundle By Name(w420) -> ("Meas start time"=w419:dbl)
        n110 = call "Read_RD_Ch_header.vi"("Raw data file"=w408) -> ("Ch Name Out"=w407:string[], "Ch Values"=w406:string[])  [unwired: 2 out]
        n111 = Search 1D Array(1D array=w407, element="Flow:Measurement:Time") -> (index of element=w416:i32)  [unwired: 1 out]
        n112 = Index Array(array=w406, index=w416) -> (element=w401:string)
        n113 = Search and Replace String(input string=w401, search string=",", replace string="." ("replace string (\"\")")) -> (result string=w402:string)  [unwired: 5 in, 3 out]
        n114 = Fract/Exp String To Number(string=w402, default (0 dbl)=nan ("default (0 DBL)")) -> (number=w399:dbl)  [unwired: 3 out]
        n115 = Not A Number/Path/Refnum?(number/path/refnum=w399) -> (NaN/Path/Refnum?=w413:bool)
        n116 = Multiply(x=w399, y=60.0) -> (x*y=w414:dbl)
        n117 = Add(x=w419, y=w414) -> (x+y=w418:dbl)
        n118 = Bundle By Name(cluster=w420, "Meas end time"=w418) -> (w423:T6)
        n119 = Select(t="Add Drift Info", s=w413, f="Get Calib Points array") -> (s? t:f=w410:string)
      }
      frame "Get Calib Points array" {
        # "Fraction = (Av_Meas_Time - Calib1_time)  /  (Calib2_time - Calib1_time)"
        n120 = Unbundle By Name(w436) -> ("Meas start time"=w441:dbl, "Meas end time"=w440:dbl, "2nd Calib time"=w442:dbl, "1st Calib time"=w431:dbl)
        n121 = Add(x=w441, y=w440) -> (x+y=w444:dbl)
        n122 = Divide(x=w444, y=2.0) -> (x/y=w439:dbl)
        n123 = Subtract(x=w442, y=w431) -> (x-y=w437:dbl)
        n124 = Subtract(x=w439, y=w431) -> (x-y=w438:dbl)
        n125 = Divide(x=w438, y=w437) -> (x/y=w435:dbl)
        n126 = case shown="\"Generic Polynomial\"" w432 {
          tunnel: ["Add Drift Info" "Single Hot wire" "Generic Polynomial" "Cross wire" w455] -> w446
          tunnel: w431 -> [_ _ _ _ w458]
          frame "Propeller anemometer", Default {
          }
          frame "Hot wire" {
          }
          frame "Generic Polynomial" {
          }
          frame "Cross wire 1" {
          }
          frame "Fast FID" {
            n127 = Not A Number/Path/Refnum?(number/path/refnum=w458) -> (NaN/Path/Refnum?=w457:bool)
            n128 = Select(t="Bkgnd info from header", s=w457, f="Fast FID") -> (s? t:f=w455:string)
          }
        }
        n129 = Bundle By Name(cluster=w436, "Fraction"=w435) -> (w434:T6)
      }
      frame "Fast FID" {
        # "Concentrations"
        # "Voltage"
        # "End"
        # "Start"
        # "(End-Start)*Fraction + Start"
        n130 = Index Array(array=w479, index (col)=1) -> (element=w486:dbl[])  [unwired: 1 in]
        n131 = call "2nd_order_Poly_convert.vi"("Calib constants"=w483, "Voltage"=w486) -> ("Eng Values"=w487:dbl[])  [unwired: 4 out]
        n132 = call "2nd_order_Poly_convert.vi"("Calib constants"=w462, "Voltage"=w486) -> ("Eng Values"=w488:dbl[])  [unwired: 4 out]
        n133 = Unbundle By Name(w481) -> ("Fraction"=w476:dbl)
        n134 = In Range and Coerce(upper limit=1.0, x=w476, lower limit=0.0) -> (coerced(x)=w473:dbl)  [unwired: 1 out]
        n135 = for {
          tunnel: w488 -> [w492] mode=indexing
          tunnel: w487 -> [w496] mode=indexing
          tunnel: w473 -> [w494]
          tunnel: [w491] -> w485 mode=indexing
          n136 = Subtract(x=w496, y=w492) -> (x-y=w495:dbl)
          n137 = Multiply(x=w494, y=w495) -> (x*y=w493:dbl)
          n138 = Add(x=w492, y=w493) -> (x+y=w491:dbl)
        }
        n139 = Index Array(array=w462, index=5) -> (element=w460:dbl)
        n140 = Format Into String(format string="Calib Fraction %.4f; ", initial string=w472, w473) -> (resulting string=w470:string)  [unwired: 1 in, 1 out]
        n141 = Build Array(w460) -> (w459:dbl[])
        n142 = call <vilib>:"General Polynomial Fit.vi"("Y"=w485, "polynomial order"=2, "X"=w486) -> ("Polynomial Coefficients"=w465:dbl[])  [unwired: 9 in, 3 out]
        n143 = call "2nd_order_Poly_convert.vi"("Calib constants"=w465, "Voltage"=w459) -> ("Eng Values"=w467:dbl[])  [unwired: 4 out]
        n144 = Index Array(array=w467) -> (element=w466:dbl)  [unwired: 1 in]
        n145 = Replace Array Subset(array=w462, new element=w465, index=0) -> (w464:dbl[])
        n146 = Replace Array Subset(array=w464, new element=w466, index=3) -> (w463:dbl[])
      }
      frame "Generic Polynomial" {
        # "Voltage"
        # "End"
        # "Start"
        # "(End-Start)*Fraction + Start"
        n147 = Index Array(array=w515, index (col)=1) -> (element=w502:dbl[])  [unwired: 1 in]
        n148 = for {
          tunnel: w502 -> [w527] mode=indexing
          tunnel: w501 -> [w526]
          tunnel: [w525] -> w500 mode=indexing
          n149 = call "Polynomial_convert.vi"("Calib constants"=w526, "Voltage"=w527) -> ("Eng Values"=w525:dbl)  [unwired: 4 in]
        }
        n150 = for {
          tunnel: w502 -> [w530] mode=indexing
          tunnel: w499 -> [w529]
          tunnel: [w528] -> w503 mode=indexing
          n151 = call "Polynomial_convert.vi"("Calib constants"=w529, "Voltage"=w530) -> ("Eng Values"=w528:dbl)  [unwired: 4 in]
        }
        n152 = for {
          tunnel: w499 -> [w524] mode=indexing
          tunnel: [w522] -> w498
          i -> [w522]
          stop <- w523 stop-if-true
          n153 = Equal To 0?(x=w524) -> (x = 0?=w523:bool)
        }
        n154 = Unbundle By Name(w517) -> ("Fraction"=w512:dbl)
        n155 = In Range and Coerce(upper limit=1.0, x=w512, lower limit=0.0) -> (coerced(x)=w509:dbl)  [unwired: 1 out]
        n156 = for {
          tunnel: w503 -> [w532] mode=indexing
          tunnel: w500 -> [w536] mode=indexing
          tunnel: w509 -> [w534]
          tunnel: [w531] -> w519 mode=indexing
          n157 = Subtract(x=w536, y=w532) -> (x-y=w535:dbl)
          n158 = Multiply(x=w534, y=w535) -> (x*y=w533:dbl)
          n159 = Add(x=w532, y=w533) -> (x+y=w531:dbl)
        }
        n160 = Format Into String(format string="Calib Fraction %.4f; ", initial string=w508, w509) -> (resulting string=w506:string)  [unwired: 1 in, 1 out]
        n161 = call <vilib>:"General Polynomial Fit.vi"("Y"=w519, "polynomial order"=w498, "X"=w502) -> ("Polynomial Coefficients"=w504:dbl[])  [unwired: 9 in, 3 out]
        n162 = Replace Array Subset(array=w499, new element=w504, index=0) -> (w497:dbl[])
      }
      frame "Single Hot wire" {
        # "U"
        # "Volts"
        n163 = Index Array(array=w541, index=7) -> (element=w547:dbl)
        n164 = Equal?(x=w547, y=w546) -> (x = y?=w545:bool)
        n165 = Index Array(array=w542, index (col)=1) -> (element=w555:dbl[])  [unwired: 1 in]
        n166 = Index Array(array=w542, index (col)=0) -> (element=w554:dbl[])  [unwired: 1 in]
        n167 = Unbundle By Name(w568) -> ("Fraction"=w564:dbl)
        n168 = In Range and Coerce(upper limit=1.0, x=w564, lower limit=0.0) -> (coerced(x)=w553:dbl)  [unwired: 1 out]
        n169 = case shown="True" w545 {
          tunnel: w541 -> [w582 w587]
          tunnel: w558 -> [w581 w596]
          tunnel: w555 -> [w580 w592]
          tunnel: w554 -> [w579 w593]
          tunnel: w553 -> [w578 w591]
          tunnel: w552 -> [w576 _]
          tunnel: w551 -> [w575 _]
          tunnel: w550 -> [w574 _]
          tunnel: w544 -> [_ w595]
          tunnel: w543 -> [w569 w594]
          tunnel: w542 -> [_ w590]
          tunnel: w541 -> [w573 _]
          tunnel: [w570 w586] -> w540
          tunnel: w539 -> [_ w585]
          tunnel: w538 -> [_ w584]
          tunnel: [w569 w583] -> w537
          frame False {
            n170 = call "SingleWire_drift_correction_PN.vi"("calib consts. t1"=w582, "Tmeas (degC)"=w576, "variable n"=w575, "calib consts. t2"=w581, "{E_cal1}"=w580, "{U_cal1}"=w579, "time fraction"=w578, "wire diameter (mu.m)"=w574) -> ("[A, B, n]"=w577:dbl[])  [unwired: 1 in, 6 out]
            n171 = Build Array (concatenate)(w577, w576) -> (w572:dbl[])
            n172 = Replace Array Subset(array=w573, new element=w572, index=0) -> (w570:dbl[])
          }
          frame True {
            n173 = Index Array(array=w590, index (col)=4 ("disabled index (col)")) -> (element=w588:dbl[])  [unwired: 1 in]
            n174 = stacked-sequence {
              seq-local: [w604 _] -> [_ w636]
              tunnel: w596 -> [w617 _]
              tunnel: w595 -> [w612 _]
              tunnel: w594 -> [w614 w626]
              tunnel: w593 -> [w609 w631]
              tunnel: w592 -> [w610 w635]
              tunnel: w591 -> [w600 _]
              tunnel: w588 -> [w608 w634]
              tunnel: w587 -> [_ w639]
              tunnel: [_ w639] -> w586
              tunnel: w585 -> [w611 _]
              tunnel: w584 -> [_ w627]
              tunnel: [_ w625] -> w583
              frame #0 {
                # "Get 2nd calibration"
                n175 = Index Array(array=w617, index #1=4 ("index"), index #2=6 ("index"), index #3=7 ("index")) -> (element #1=w620:dbl, element #2=w602:dbl, element #3=w601:dbl)
                n176 = Increment(x=w620) -> (x+1=w603:dbl)
                n177 = Concatenate Strings(w611, w612) -> (w615:string)
                n178 = call "2D_array_from_string.vi"("Show Dialog?"=FALSE, "Input string"=w614, "Array title"=w615) -> ("2D data array"=w613:dbl[][])  [unwired: 1 in]
                n179 = Index Array(array=w613, index (col)=0 ("disabled index (col)")) -> (element=w606:dbl[])  [unwired: 1 in]
                n180 = Index Array(array=w613, index (col)=4 ("disabled index (col)")) -> (element=w605:dbl[])  [unwired: 1 in]
                n181 = Index Array(array=w613, index (col)=1 ("disabled index (col)")) -> (element=w607:dbl[])  [unwired: 1 in]
                n182 = call "Example virtual calibration data generator.vi"("t0_U_cal t0 (m/s)"=w609, "t0_Vout_cal t0 (V)"=w610, "time fraction (0...1)"=w600, "t0_Ta_cal (°C)"=w608, "t1_Vout_cal t0 (V)"=w607, "t1_U_cal t0 (m/s)"=w606, "t1_Ta_cal (°C)"=w605, "Overheat ratio"=w603, "Gain"=w602, "Offset (V)"=w601) -> ("t_frac Calibration data"=w597:T8, "t1* Calibration data"=w604:T8)  [unwired: 3 in, 1 out]
                n183 = global read "CTA Calib Coeff Global.vi" "HW Calibration Cluster"() -> (w599:T8[])
                n184 = Build Array (concatenate)(w599, w597) -> (w598:T8[])
                n185 = global write "CTA Calib Coeff Global.vi" "HW Calibration Cluster"(w598) -> ()
              }
              frame #1 {
                n186 = Index Array(array=w639, index #1=4 ("index"), index #2=6 ("index"), index #3=7 ("index")) -> (element #1=w641:dbl, element #2=w638:dbl, element #3=w637:dbl)
                n187 = Increment(x=w641) -> (x+1=w640:dbl)
                n188 = for {
                  tunnel: w636 -> [w651]
                  tunnel: w635 -> [w650] mode=indexing
                  tunnel: w634 -> [w649] mode=indexing
                  tunnel: w640 -> [w648]
                  tunnel: w638 -> [w647]
                  tunnel: w637 -> [w646]
                  tunnel: [w645] -> w633 mode=indexing
                  n189 = call "Example data post-processing (single point).vi"("Calibration data"=w651, "V_out (V)"=w650, "Ta (°C)"=w649, "Overheat ratio (Rw / R0)"=w648, "Gain"=w647, "Offset (V)"=w646) -> ("U (m/s)"=w645:dbl)  [unwired: 9 in]
                }
                n190 = Build Array(w633, w631) -> (w632:dbl[][])
                n191 = call "Calib_Change.vi"("Eng Units"=w632) -> ("% Change"=w630:dbl)
                n192 = Number To Fractional String(number=w630, precision (6)=i16 2) -> (F-format string=w628:string)  [unwired: 2 in]
                n193 = call "Replace_data_in_setup_string.vi"("New data string"=w628, "Input string"=w626, "Variable name"=w627) -> ("Appended string"=w625:string)
              }
            }
          }
        }
        n194 = Format Into String(format string="Calib Fraction %.4f; ", initial string=w561, w553) -> (resulting string=w559:string)  [unwired: 1 in, 1 out]
      }
      frame "Cross wire" {
        n195 = for {
          tunnel: w681 -> [w738]
          tunnel: w682 -> [w737]
          tunnel: [w736] -> w675 mode=indexing
          tunnel: [w735] -> w674 mode=indexing
          tunnel: i32[] [0, 1, 2, 9, 10, 12, 14, 15] -> [w734] mode=indexing
          n196 = Index Array(array=w738, index=w734) -> (element=w736:dbl)
          n197 = Index Array(array=w737, index=w734) -> (element=w735:dbl)
        }
        n198 = for {
          tunnel: i32[] [3, 4, 5, 9, 11, 13, 16, 17] -> [w733] mode=indexing
          tunnel: w682 -> [w732]
          tunnel: [w731] -> w667 mode=indexing
          tunnel: w681 -> [w730]
          tunnel: [w729] -> w668 mode=indexing
          n199 = Index Array(array=w730, index=w733) -> (element=w729:dbl)
          n200 = Index Array(array=w732, index=w733) -> (element=w731:dbl)
        }
        n201 = Index Array(array=w671, index (col)=1) -> (element=w673:dbl[])  [unwired: 1 in]
        n202 = Index Array(array=w671, index (col)=0) -> (element=w670:dbl[])  [unwired: 1 in]
        n203 = Index Array(array=w671, index (col)=2) -> (element=w669:dbl[])  [unwired: 1 in]
        n204 = Unbundle By Name(w695) -> ("Fraction"=w691:dbl)
        n205 = In Range and Coerce(upper limit=1.0, x=w691, lower limit=0.0) -> (coerced(x)=w666:dbl)  [unwired: 1 out]
        n206 = call "SingleWire_drift_correction_PN.vi"("calib consts. t1"=w675, "Tmeas (degC)"=w662, "variable n"=w663, "calib consts. t2"=w674, "{E_cal1}"=w673, "{U_cal1}"=w670, "time fraction"=w666, "wire diameter (mu.m)"=w661) -> ("[A, B, n]"=w665:dbl[])  [unwired: 1 in, 6 out]
        n207 = call "SingleWire_drift_correction_PN.vi"("calib consts. t1"=w668, "Tmeas (degC)"=w662, "variable n"=w663, "calib consts. t2"=w667, "{E_cal1}"=w669, "{U_cal1}"=w670, "time fraction"=w666, "wire diameter (mu.m)"=w661) -> ("[A, B, n]"=w664:dbl[])  [unwired: 1 in, 6 out]
        n208 = Replace Array Subset(array=w681, new element=w662, index=9) -> (w677:dbl[])
        n209 = Replace Array Subset(array=w677, new element=w665, index=0) -> (w676:dbl[])
        n210 = Replace Array Subset(array=w676, new element=w664, index=3) -> (w657:dbl[])
        n211 = Format Into String(format string="Calib Fraction %.4f; ", initial string=w688, w666) -> (resulting string=w686:string)  [unwired: 1 in, 1 out]
        n212 = case shown="False" w659 {
          tunnel: w660 -> [w704 _]
          tunnel: w658 -> [w698 _]
          tunnel: w657 -> [w703 _]
          tunnel: w656 -> [w702 _]
          tunnel: w655 -> [w701 _]
          tunnel: w654 -> [w700 _]
          tunnel: w653 -> [w699 _]
          frame False {
            n213 = case shown="\"Triangle mesh\", \"Polynomial surface\"" w698 {
              selector: w698 -> [w712 _ _]
              tunnel: w704 -> [w706 _ _]
              tunnel: w703 -> [w717 _ _]
              tunnel: w702 -> [w716 _ _]
              tunnel: w701 -> [w715 _ _]
              tunnel: w700 -> [w714 _ _]
              tunnel: w699 -> [w713 _ _]
              frame "Triangle mesh", "Polynomial surface" {
                n214 = call "Get Raw Data Folder.vi"("Raw data file"=w706) -> ("Main Raw Data Folder"=w705:path)
                n215 = Build Path(base path=w705, name or relative path="XW_Map.txt") -> (appended path=w718:path)
                n216 = Build Path(base path=w705, name or relative path="XW_Map_CALPTS.txt") -> (appended path=w711:path)
                n217 = call "Does_file_exist_(simple).vi"("Pathname"=w718) -> ("exists?"=w708:bool)
                n218 = call "Does_file_exist_(simple).vi"("Pathname"=w711) -> ("exists?"=w709:bool)
                n219 = And(x=w708, y=w709) -> (x .and. y?=w707:bool)
                n220 = case shown="True" w707 {
                  tunnel: w718 -> [_ w726]
                  tunnel: w712 -> [_ w727]
                  tunnel: w717 -> [_ w725]
                  tunnel: w716 -> [_ w724]
                  tunnel: w715 -> [_ w723]
                  tunnel: w714 -> [_ w722]
                  tunnel: w713 -> [_ w721]
                  frame False {
                    n221 = global write "XW_Map_Global.vi" "Map method"(Map_method."Const. Psi_eff (std.)" ("Map method")) -> ()
                  }
                  frame True {
                    n222 = call "XW_Map_PreProc_wrapper_PN.vi"("Domain padding factor"=w721, "cap indicial sum to n"=w722, "XW_Calib_Map file path"=w726, "surface order (n)"=w723, "Apply calibration corrections"=w724, "Calib const"=w725, "Map method"=w727) -> ()  [unwired: 5 out]
                  }
                }
              }
              frame "Psi_eff = f(Umagn.)", "Psi_eff, k = f(Umagn.)" {
              }
              frame "Const. Psi_eff (std.)" {
                n223 = global write "XW_Map_Global.vi" "Map method"(Map_method."Const. Psi_eff (std.)" ("Map method")) -> ()
              }
            }
          }
          frame True {
          }
        }
      }
      frame "Bkgnd info from header" {
        # "After"
        # "Before"
        # "Start"
        # "end"
        n224 = stacked-sequence {
          seq-local: [w758 _ _ _ _ _ _] -> [_ _ w779 _ w900 _ _]
          seq-local: [w760 _ _ _ _ _ _] -> [_ _ w777 _ w892 _ _]
          seq-local: [w759 _ _ _ _ _ _] -> [_ _ w776 _ w903 _ _]
          seq-local: [_ w767 _ _ _ _ _] -> [_ _ w775 _ w901 w1095 _]
          seq-local: [_ _ w774 _ _ _ _] -> [_ _ _ _ w898 _ _]
          seq-local: [_ _ w773 _ _ _ _] -> [_ _ _ w889 w902 w1096 _]
          seq-local: [_ _ w772 _ _ _ _] -> [_ _ _ w890 _ w1097 _]
          seq-local: [_ _ _ w875 _ _ _] -> [_ _ _ _ w905 _ _]
          seq-local: [_ _ _ w884 _ _ _] -> [_ _ _ _ _ w1098 _]
          seq-local: [_ _ _ _ w895 _ _] -> [_ _ _ _ _ w1092 _]
          tunnel: w757 -> [w761 w766 _ _ _ _ _]
          tunnel: w756 -> [_ _ w778 _ w893 _ _]
          tunnel: w755 -> [_ w762 _ w891 _ w1094 _]
          tunnel: [_ w766 _ _ _ _ _] -> w754
          tunnel: w753 -> [_ w765 _ _ _ _ _]
          tunnel: [_ w765 _ _ _ _ _] -> w752
          tunnel: [_ w764 _ _ _ _ _] -> w751
          tunnel: w750 -> [_ w764 _ _ _ _ _]
          tunnel: w749 -> [_ _ _ _ w899 w1093 _]
          tunnel: [_ _ _ _ _ w1091 _] -> w748
          tunnel: [_ w763 _ _ _ _ _] -> w747
          tunnel: w746 -> [_ w763 _ _ _ _ _]
          tunnel: [_ _ _ _ _ _ w1157] -> w745
          tunnel: [_ _ _ _ TRUE _ _] -> w744
          tunnel: [_ w762 _ _ _ _ _] -> w743
          tunnel: [_ _ _ _ w896 _ _] -> w742
          tunnel: w741 -> [_ _ _ _ w897 _ _]
          tunnel: w739 -> [_ _ _ _ w904 _ w1159]
          frame #0 {
            n225 = call "Read FFID_Header.vi"("Raw Data header String"=w761) -> ("Ch names"=w760:string[], "FFID Header Info"=w759:string[][], "Bkgnd Volts Present?"=w758:bool)
            "Header info" <- w759
          }
          frame #1 {
            n226 = Unbundle By Name(w762) -> ("Meas start time"=w771:dbl, "Meas end time"=w770:dbl)
            n227 = Add(x=w771, y=w770) -> (x+y=w769:dbl)
            n228 = Divide(x=w769, y=2.0) -> (x/y=w767:dbl)
          }
          frame #2 {
            n229 = case shown="True" w779 {
              tunnel: w778 -> [w797 w851]
              tunnel: w777 -> [w784 w841]
              tunnel: w776 -> [w786 w842]
              tunnel: w775 -> [w783 _]
              tunnel: [w782 w828] -> w774
              tunnel: [w781 w828] -> w773
              tunnel: [w780 w828] -> w772
              frame True {
                n230 = Decimal String To Number(string=w797) -> (number=w796:i32)  [unwired: 3 out]
                n231 = Index Array(array=w786, index (col)=0 ("disabled index (col)")) -> (element=w791:string[])  [unwired: 1 in]
                n232 = Number To Decimal String(number=w796) -> (decimal integer string=w795:string)  [unwired: 1 out]
                n233 = Search 1D Array(1D array=w791, element="Calibration Before Meas") -> (index of element=w789:i32)  [unwired: 1 out]
                n234 = Search 1D Array(1D array=w791, element="Calibration After Meas") -> (index of element=w787:i32)  [unwired: 1 out]
                n235 = Index Array(array=w786, index (row)=w789) -> (element=w788:string[])  [unwired: 1 in]
                n236 = Index Array(array=w786, index (row)=w787) -> (element=w785:string[])  [unwired: 1 in]
                n237 = for {
                  tunnel: w795 -> [w813]
                  tunnel: string[] ["Bkgnd Time", "Bkgnd Volts", "Bkgnd Variance"] ("appended array") -> [w812] mode=indexing
                  tunnel: w788 -> [w811]
                  tunnel: w785 -> [w809]
                  tunnel: w784 -> [w807]
                  tunnel: w783 -> [w805]
                  shift-right: [w801] -> _
                  shift-left: _ -> [w802]
                  tunnel: [w800] -> w782 mode=indexing
                  tunnel: [w799] -> w781 mode=indexing
                  tunnel: [w798] -> w780 mode=indexing
                  i -> [w806]
                  # "After"
                  # "Before"
                  n238 = Concatenate Strings("FF:", w813, ":" ("Substring"), w812) -> (w814:string)
                  n239 = Search 1D Array(1D array=w807, element=w814) -> (index of element=w810:i32)  [unwired: 1 out]
                  n240 = Index Array(array=w811, index=w810) -> (element=w804:string)
                  n241 = Index Array(array=w809, index=w810) -> (element=w803:string)
                  n242 = call "String_2_Number.vi"("Value"=w804) -> ("Numeric"=w799:dbl)
                  n243 = call "String_2_Number.vi"("Value"=w803) -> ("Numeric"=w798:dbl)
                  n244 = case shown="1, Default" w806 {
                    tunnel: w805 -> [w821 _]
                    tunnel: w799 -> [w819 w824]
                    tunnel: w798 -> [w820 w827]
                    tunnel: [w816 w823] -> w800
                    tunnel: w802 -> [_ w822]
                    tunnel: [w816 w822] -> w801
                    frame 0 {
                      n245 = Subtract(x=w821, y=w819) -> (x-y=w817:dbl)
                      n246 = Subtract(x=w820, y=w819) -> (x-y=w818:dbl)
                      n247 = Divide(x=w817, y=w818) -> (x/y=w816:dbl)
                    }
                    frame 1, Default {
                      n248 = Subtract(x=w827, y=w824) -> (x-y=w826:dbl)
                      n249 = Multiply(x=w822, y=w826) -> (x*y=w825:dbl)
                      n250 = Add(x=w825, y=w824) -> (x+y=w823:dbl)
                    }
                  }
                }
              }
              frame False {
                n251 = Decimal String To Number(string=w851) -> (number=w850:i32)  [unwired: 3 out]
                n252 = Index Array(array=w842, index (col)=0 ("disabled index (col)")) -> (element=w845:string[])  [unwired: 1 in]
                n253 = Number To Decimal String(number=w850) -> (decimal integer string=w849:string)  [unwired: 1 out]
                n254 = Search 1D Array(1D array=w845, element="Calibration To be Used") -> (index of element=w844:i32)  [unwired: 1 out]
                n255 = Index Array(array=w842, index (row)=w844) -> (element=w843:string[])  [unwired: 1 in]
                n256 = for {
                  tunnel: w849 -> [w872]
                  tunnel: string[] ["Coeff A", "Coeff B", "Coeff C", "Bkgnd", "Bkgnd Variance"] ("appended array") -> [w871] mode=indexing
                  tunnel: w843 -> [w870]
                  tunnel: w841 -> [w868]
                  tunnel: [w866] -> w831 mode=indexing
                  tunnel: [w865] -> w834 mode=indexing
                  n257 = Concatenate Strings("FF:", w872, ":" ("Substring"), w871) -> (w873:string)
                  n258 = Search 1D Array(1D array=w868, element=w873) -> (index of element=w865:i32)  [unwired: 1 out]
                  n259 = Index Array(array=w870, index=w865) -> (element=w867:string)
                  n260 = call "String_2_Number.vi"("Value"=w867) -> ("Numeric"=w866:dbl)
                }
                n261 = Index Array(array=w831, index=3 ("length")) -> (element=w839:dbl)
                n262 = Index Array(array=w831, index=4) -> (element=w836:dbl)
                n263 = Index Array(array=w834, index=2) -> (element=w832:i32)
                n264 = Less Than 0?(x=w832) -> (x < 0?=w830:bool)
                n265 = case shown="False" w830 {
                  tunnel: w831 -> [w853 w859]
                  tunnel: [w852 w855] -> w829
                  frame False {
                    n266 = Array Subset(array=w853, length=3) -> (w852:dbl[])  [unwired: 1 in]
                  }
                  frame True {
                    n267 = Index Array(array=w859, index=1) -> (element=w863:dbl)
                    n268 = Index Array(array=w859, index=0) -> (element=w862:dbl)
                    n269 = Reciprocal(x=w863) -> (1/x=w857:dbl)
                    n270 = Divide(x=w862, y=w863) -> (x/y=w864:dbl)
                    n271 = Negate(x=w864) -> (-x=w858:dbl)
                    n272 = Build Array(w858, w857, 0.0 ("element")) -> (w855:dbl[])
                  }
                }
                n273 = call "Polybackwards.vi"("Coefficients"=w829, "Y input"=w839) -> ("X output"=w837:dbl)  [unwired: 1 out]
                n274 = Build Array(0.0 ("element"), w837, w836) -> (w828:dbl[])
              }
            }
          }
          frame #3 {
            # "Bkgnd Time"
            n275 = Unbundle By Name(w891) -> ("1st Calib time"=w883:dbl, "2nd Calib time"=w878:dbl)
            n276 = Index Array(array=w890) -> (element #1=w879:dbl, element #2=w881:dbl)  [unwired: 2 in]
            n277 = Index Array(array=w889) -> (element #1=w888:dbl, element #2=w882:dbl)  [unwired: 2 in]
            n278 = Greater?(x=w879, y=w878) -> (0:w876:bool)
            n279 = Greater Than 0?(x=w878) -> (x > 0?=w877:bool)
            n280 = Greater?(x=w882, y=w881) -> (0:w885:bool)
            n281 = And(x=w876, y=w877) -> (x .and. y?=w875:bool)
            n282 = Subtract(x=w888, y=w883) -> (x-y=w880:dbl)
            n283 = Less?(x=w880, y=250.0) -> (x < y?=w886:bool)
            n284 = And(x=w886, y=w885) -> (x .and. y?=w884:bool)
          }
          frame #4 {
            n285 = case shown="True" w905 {
              tunnel: w904 -> [_ w969]
              tunnel: w903 -> [_ w968]
              tunnel: w902 -> [w913 w959]
              tunnel: w901 -> [_ w967]
              tunnel: w900 -> [w912 _]
              tunnel: w899 -> [w911 w964]
              tunnel: w898 -> [w910 w966]
              tunnel: w897 -> [w909 w963]
              tunnel: [w908 w962] -> w896
              tunnel: [w907 w965] -> w895
              tunnel: w893 -> [_ w961]
              tunnel: w892 -> [_ w960]
              frame False {
                n286 = Index Array(array=w910, index=1) -> (element=w915:dbl)
                n287 = Index Array(array=w910, index=2) -> (element=w922:dbl)
                n288 = Build Array(w915) -> (w914:dbl[])
                n289 = Index Array(array=w913) -> (element #1=w918:dbl, element #2=w917:dbl, element #3=w916:dbl)  [unwired: 3 in]
                n290 = Index Array(array=w910, index=0) -> (element=w920:dbl)
                n291 = call "2nd_order_Poly_convert.vi"("Calib constants"=w911, "Voltage"=w914) -> ("Eng Values"=w927:dbl[])  [unwired: 4 out]
                n292 = Not A Number/Path/Refnum?(number/path/refnum=w910) -> (NaN/Path/Refnum?=w919:bool[])
                n293 = Or Array Elements(Boolean array=w919) -> (logical OR=w906:bool)
                n294 = Index Array(array=w927, index=0) -> (element=w923:dbl)
                n295 = case shown="False" w906 {
                  tunnel: w911 -> [w945 w957]
                  tunnel: w923 -> [w943 _]
                  tunnel: w922 -> [w940 _]
                  tunnel: [w931 w957] -> w907
                  tunnel: w920 -> [w938 _]
                  tunnel: [w935 w958] -> w908
                  tunnel: w909 -> [w934 w958]
                  tunnel: w912 -> [w928 _]
                  tunnel: w918 -> [w933 _]
                  tunnel: w917 -> [w930 _]
                  tunnel: w916 -> [w929 _]
                  frame False {
                    n296 = Equal To 0?(x=w938) -> (x = 0?=w937:bool)
                    n297 = Replace Array Subset(array=w945, new element=w943, index=3) -> (w942:dbl[])
                    n298 = Format Into String(format string="Bkgnd Fraction %.4f; ", initial string=w934, w938) -> (resulting string=w936:string)  [unwired: 1 in, 1 out]
                    n299 = Replace Array Subset(array=w942, new element=w940, index=4) -> (w932:dbl[])
                    n300 = case shown="True" w928 {
                      tunnel: w933 -> [_ w956]
                      tunnel: w932 -> [w946 w955]
                      tunnel: [w946 w950] -> w931
                      tunnel: w930 -> [_ w949]
                      tunnel: w929 -> [_ w948]
                      frame False {
                      }
                      frame True {
                        n301 = Replace Array Subset(array=w955, new element=w956, index=8) -> (w952:dbl[])
                        n302 = Replace Array Subset(array=w952, new element=w949, index=9) -> (w951:dbl[])
                        n303 = Replace Array Subset(array=w951, new element=w948, index=10) -> (w950:dbl[])
                      }
                    }
                    n304 = Select(t=w934, s=w937, f=w936) -> (s? t:f=w935:string)
                  }
                  frame True {
                  }
                }
              }
              frame True {
                # "File"
                # "Time"
                # "Volts"
                n305 = stacked-sequence {
                  seq-local: [_ w988 _ _] -> [_ _ w1068 _]
                  seq-local: [_ w987 _ _] -> [_ _ w1067 _]
                  seq-local: [_ w986 _ _] -> [_ _ _ w1077]
                  seq-local: [_ _ w1048 _] -> [_ _ _ w1072]
                  seq-local: [w974 _ _ _] -> [_ w985 _ _]
                  seq-local: [w970 _ _ _] -> [_ w984 _ _]
                  tunnel: w969 -> [_ w1005 _ _]
                  tunnel: w968 -> [_ w991 _ w1079]
                  tunnel: w959 -> [_ _ w1066 _]
                  tunnel: w967 -> [_ _ w1051 _]
                  tunnel: w966 -> [_ _ _ _]
                  tunnel: [_ _ _ w1075] -> w965
                  tunnel: w964 -> [_ _ w1054 w1076]
                  tunnel: w963 -> [_ _ _ w1074]
                  tunnel: [_ _ _ w1073] -> w962
                  tunnel: w961 -> [w977 _ _ _]
                  tunnel: w960 -> [w971 _ _ _]
                  frame #0 {
                    n306 = Decimal String To Number(string=w977) -> (number=w978:i32)  [unwired: 3 out]
                    n307 = Number To Decimal String(number=w978) -> (decimal integer string=w975:string)  [unwired: 1 out]
                    n308 = for {
                      tunnel: string[] ["Calib Filename", "Bkgnd Volts", "Bkgnd Time"] ("appended array") -> [w981] mode=indexing
                      tunnel: w975 -> [w980]
                      tunnel: [w979] -> w974 mode=indexing
                      n309 = Concatenate Strings("FF:", w980, ":" ("Substring"), w981) -> (w979:string)
                    }
                    n310 = Index Array(array=w974, index=2) -> (element=w972:string)
                    n311 = Search 1D Array(1D array=w971, element=w972) -> (index of element=w970:i32)  [unwired: 1 out]
                  }
                  frame #1 {
                    w997 = "_" ("regular expression")
                    n312 = Index Array(array=w991, index (row)=0, index (col)=w984) -> (element=w990:string)
                    n313 = Strip Path(path=w1005) -> (stripped path=w989:path, name=w1004:string)
                    n314 = Reverse String(1:w1004) -> (0:w1003:string)
                    n315 = Match Pattern(string=w1003, regular expression=w997) -> (before substring=w1002:string, after substring=w999:string)  [unwired: 1 in, 2 out]
                    n316 = Reverse String(1:w1002) -> (0:w1000:string)
                    n317 = Reverse String(1:w999) -> (0:w998:string)
                    n318 = Decimal String To Number(string=w1000) -> (offset past number=w1001:i32, number=w994:i32)  [unwired: 2 in]
                    n319 = Decrement(x=w994) -> (x-1=w993:i32)
                    n320 = String Subset(string=w1000, offset (0)=w1001) -> (substring=w996:string)  [unwired: 1 in]
                    n321 = for {
                      N: 20 -> [_]
                      tunnel: w998 -> [w1023]
                      tunnel: w997 -> [w1022]
                      tunnel: w996 -> [w1020]
                      tunnel: w993 -> [w1018]
                      tunnel: w990 -> [w1006]
                      tunnel: w989 -> [w1017]
                      tunnel: [w1013] -> w988
                      tunnel: [w1012] -> w987
                      tunnel: [w1014] -> w986
                      tunnel: w985 -> [w1015]
                      i -> [w1019]
                      stop <- w1007 continue-if-true
                      n322 = Subtract(x=w1018, y=w1019) -> (x-y=w1011:i32)
                      n323 = Equal To 0?(x=w1011) -> (x = 0?=w1010:bool)
                      n324 = Number To Decimal String(number=w1011) -> (decimal integer string=w1021:string)  [unwired: 1 in]
                      n325 = Concatenate Strings(w1023, w1022, w1021, w1020) -> (w1016:string)
                      "Earlier raw data file" <- w1016
                      n326 = case shown="True" w1010 {
                        tunnel: w1017 -> [w1035 _]
                        tunnel: w1016 -> [w1034 _]
                        tunnel: w1015 -> [w1032 _]
                        tunnel: [w1029 w1047] -> w1014
                        tunnel: [w1028 w1047] -> w1013
                        tunnel: [w1027 w1045] -> w1012
                        tunnel: [TRUE FALSE] -> w1008
                        tunnel: w1006 -> [_ w1045]
                        frame False {
                          w1037 = FALSE  # Show Dialog?
                          n327 = Build Path(base path=w1035, name or relative path=w1034) -> (appended path=w1026:path)
                          n328 = call "Read Characters with check.vi"("file (use dialog)"=w1026) -> ("Read String"=w1025:string)  [unwired: 1 in, 1 out]
                          n329 = call "Get_string_subset.vi"("Show Dialog?"=w1037, "String to split"=w1025, "File Label"="Raw data header") -> ("Output string"=w1036:string)  [unwired: 1 in, 1 out]
                          n330 = call "Read FFID_Header.vi"("Raw Data header String"=w1036) -> ("Ch names"=w1033:string[], "FFID Header Info"=w1031:string[][])  [unwired: 1 out]
                          n331 = for {
                            tunnel: [w1043] -> w1030 mode=indexing
                            tunnel: w1033 -> [w1042]
                            tunnel: w1032 -> [w1040] mode=indexing
                            tunnel: w1031 -> [w1039]
                            n332 = Search 1D Array(1D array=w1042, element=w1040) -> (index of element=w1041:i32)  [unwired: 1 out]
                            n333 = Index Array(array=w1039, index (row)=0, index (col)=w1041) -> (element=w1043:string)
                          }
                          n334 = Index Array(array=w1030) -> (element #1=w1029:string, element #2=w1028:string, element #3=w1027:string)  [unwired: 3 in]
                        }
                        frame True {
                          w1047 = ""
                        }
                      }
                      n335 = Equal?(x=w1012, y=w1006) -> (x = y?=w1009:bool)
                      n336 = And(x=w1008, y=w1009) -> (x .and. y?=w1007:bool)
                    }
                  }
                  frame #2 {
                    n337 = Index Array(array=w1066) -> (element #1=w1065:dbl, element #2=w1063:dbl)  [unwired: 2 in]
                    n338 = Fract/Exp String To Number(string=w1068) -> (number=w1064:dbl)  [unwired: 3 in, 1 out]
                    "Volts" <- w1064
                    n339 = Fract/Exp String To Number(string=w1067) -> (number=w1050:dbl)  [unwired: 3 in, 1 out]
                    "Time" <- w1050
                    n340 = Build Array(w1050, w1065) -> (w1053:dbl[])
                    n341 = Subtract(x=w1053, y=w1050) -> (x-y=w1052:dbl[])
                    n342 = Build Array(w1064, w1063) -> (w1062:dbl[])
                    n343 = Subtract(x=w1051, y=w1050) -> (x-y=w1049:dbl)
                    n344 = call <vilib>:"Linear Fit.vi"("Y"=w1062, "X"=w1052) -> ("slope"=w1061:dbl, "intercept"=w1059:dbl)  [unwired: 9 in, 3 out]
                    n345 = Multiply(x=w1049, y=w1061) -> (x*y=w1060:dbl)
                    n346 = Add(x=w1060, y=w1059) -> (x+y=w1055:dbl)
                    n347 = Build Array(w1055) -> (w1056:dbl[])
                    n348 = call "2nd_order_Poly_convert.vi"("Calib constants"=w1054, "Voltage"=w1056) -> ("Eng Values"=w1058:dbl[])  [unwired: 4 out]
                    n349 = Index Array(array=w1058, index=0) -> (element=w1048:dbl)
                  }
                  frame #3 {
                    n350 = Not A Number/Path/Refnum?(number/path/refnum=w1072) -> (NaN/Path/Refnum?=w1071:bool)
                    n351 = Index Array(array=w1079, index (row)=0, index (col)=1 ("disabled index (col)")) -> (element=w1078:string)
                    n352 = Equal?(x=w1077, y=w1078) -> (x = y?=w1070:bool)
                    n353 = Compound Arithmetic op=AND(w1070, invert w1071) -> (w1069:bool)
                    n354 = case shown="True" w1069 {
                      tunnel: w1076 -> [w1083 w1089]
                      tunnel: [w1083 w1088] -> w1075
                      tunnel: w1074 -> [w1082 w1087]
                      tunnel: [w1082 w1086] -> w1073
                      tunnel: w1072 -> [_ w1084]
                      frame False {
                      }
                      frame True {
                        n355 = Replace Array Subset(array=w1089, new element=w1084, index=3) -> (w1088:dbl[])
                        n356 = Concatenate Strings(w1087, "Bkgnd Extrapolated;" ("string")) -> (w1086:string)
                      }
                    }
                  }
                }
              }
            }
          }
          frame #5 {
            n357 = case shown="False" w1098 {
              tunnel: w1097 -> [_ w1112]
              tunnel: w1096 -> [_ w1111]
              tunnel: w1095 -> [_ w1105]
              tunnel: w1094 -> [_ w1104]
              tunnel: w1093 -> [_ w1102]
              tunnel: w1092 -> [w1099 w1101]
              tunnel: [w1099 w1100] -> w1091
              frame False {
              }
              frame True {
                w1108 = 350.0  # Time Constant
                # "Offset"
                # "A"
                # "B2"
                # "B1"
                # "T2"
                # "T1"
                # "Ratio 2"
                # "Ratio 1"
                n358 = Unbundle By Name(w1104) -> ("1st Calib time"=w1103:dbl)
                n359 = Index Array(array=w1112) -> (element #1=w1109:dbl, element #2=w1106:dbl)  [unwired: 2 in]
                n360 = Index Array(array=w1111) -> (element #1=w1110:dbl, element #2=w1107:dbl)  [unwired: 2 in]
                n361 = stacked-sequence {
                  seq-local: [w1123 _ _ _ _] -> [_ w1129 _ _ _]
                  seq-local: [w1121 _ _ _ _] -> [_ w1128 w1134 _ _]
                  seq-local: [_ w1125 _ _ _] -> [_ _ w1133 w1140 _]
                  seq-local: [_ _ w1135 _ _] -> [_ _ _ w1138 _]
                  seq-local: [_ _ _ w1137 _] -> [_ _ _ _ w1152]
                  tunnel: w1110 -> [w1117 _ _ _ _]
                  tunnel: w1109 -> [w1114 _ _ _ _]
                  tunnel: w1108 -> [w1118 _ _ w1145 _]
                  tunnel: w1107 -> [_ w1131 _ _ _]
                  tunnel: w1106 -> [_ w1130 w1136 _ _]
                  tunnel: w1105 -> [_ _ _ w1143 _]
                  tunnel: w1103 -> [w1115 _ _ w1144 _]
                  tunnel: w1102 -> [_ _ _ _ w1151]
                  tunnel: w1101 -> [_ _ _ _ w1150]
                  tunnel: [_ _ _ _ w1149] -> w1100
                  frame #0 {
                    n362 = Subtract(x=w1117, y=w1115) -> (x-y=w1116:dbl)
                    n363 = Subtract(x=w1114, y=w1115) -> (x-y=w1113:dbl)
                    n364 = Divide(x=w1116, y=w1118) -> (x/y=w1124:dbl)
                    n365 = Divide(x=w1113, y=w1118) -> (x/y=w1122:dbl)
                    n366 = Negate(x=w1124) -> (-x=w1120:dbl)
                    n367 = Negate(x=w1122) -> (-x=w1119:dbl)
                    n368 = Exponential(1:w1120) -> (0:w1123:dbl)
                    n369 = Exponential(1:w1119) -> (0:w1121:dbl)
                  }
                  frame #1 {
                    n370 = Subtract(x=w1129, y=w1128) -> (x-y=w1126:dbl)
                    n371 = Subtract(x=w1131, y=w1130) -> (x-y=w1127:dbl)
                    n372 = Divide(x=w1127, y=w1126) -> (x/y=w1125:dbl)
                  }
                  frame #2 {
                    n373 = Multiply(x=w1134, y=w1133) -> (x*y=w1132:dbl)
                    n374 = Subtract(x=w1136, y=w1132) -> (x-y=w1135:dbl)
                  }
                  frame #3 {
                    n375 = Subtract(x=w1143, y=w1144) -> (x-y=w1142:dbl)
                    n376 = Divide(x=w1142, y=w1145) -> (x/y=w1146:dbl)
                    n377 = Negate(x=w1146) -> (-x=w1147:dbl)
                    n378 = Exponential(1:w1147) -> (0:w1141:dbl)
                    n379 = Multiply(x=w1140, y=w1141) -> (x*y=w1139:dbl)
                    n380 = Add(x=w1139, y=w1138) -> (x+y=w1137:dbl)
                  }
                  frame #4 {
                    n381 = Build Array(w1152) -> (w1156:dbl[])
                    n382 = call "2nd_order_Poly_convert.vi"("Calib constants"=w1151, "Voltage"=w1156) -> ("Eng Values"=w1155:dbl[])  [unwired: 4 out]
                    n383 = Index Array(array=w1155, index=0) -> (element=w1148:dbl)
                    n384 = Replace Array Subset(array=w1150, new element=w1148, index=3) -> (w1149:dbl[])
                  }
                }
              }
            }
          }
          frame #6 {
            n385 = Strip Path(path=w1159) -> (stripped path=w1163:path)  [unwired: 1 out]
            n386 = Build Path(base path=w1163, name or relative path="Background_History.xls") -> (appended path=w1162:path)
            n387 = call "Does_file_exist_(simple).vi"("Pathname"=w1162) -> ("exists?"=w1161:bool)
            n388 = Select(t="Bkgnd info from table", s=w1161, f="Add FFID Bkgnd Values") -> (s? t:f=w1157:string)
          }
        }
      }
      frame "Bkgnd info from table" {
        n389 = stacked-sequence {
          seq-local: [w1199 _] -> [_ w1213]
          seq-local: [_ w1204] -> [_ _]
          seq-local: [w1200 _] -> [_ w1227]
          seq-local: [w1198 _] -> [_ w1206]
          tunnel: w1183 -> [_ w1235]
          tunnel: w1182 -> [_ w1230]
          tunnel: w1181 -> [_ w1231]
          tunnel: [_ w1235] -> w1180
          tunnel: w1179 -> [_ w1234]
          tunnel: [_ w1234] -> w1178
          tunnel: [_ w1233] -> w1177
          tunnel: w1176 -> [_ w1233]
          tunnel: w1175 -> [_ w1219]
          tunnel: [_ w1209] -> w1174
          tunnel: [_ w1232] -> w1173
          tunnel: w1172 -> [_ w1232]
          tunnel: [_ "Add FFID Bkgnd Values"] -> w1171
          tunnel: [_ TRUE] -> w1170
          tunnel: [_ w1231] -> w1169
          tunnel: w1168 -> [_ w1215]
          tunnel: [_ w1214] -> w1167
          tunnel: w1165 -> [_ w1204]
          frame #0 {
            n390 = global read "Meas_global.vi" "Raw data file"() -> (w1197:path)
            n391 = Strip Path(path=w1197) -> (stripped path=w1195:path)  [unwired: 1 out]
            n392 = Build Path(base path=w1195, name or relative path="Background_History.xls") -> (appended path=w1185:path)
            n393 = call "Read Characters with check.vi"("file (use dialog)"=w1185) -> ("Read String"=w1184:string)  [unwired: 1 in, 1 out]
            n394 = call "String_to_Ch_names.vi"("Spreadsheet string"=w1184) -> ("Ch names"=w1187:string[], "String After names"=w1192:string)  [unwired: 2 out]
            n395 = Spreadsheet String To Array(format string="%s", spreadsheet string=w1192, array type (2D Dbl)=string[][] []) -> (array=w1189:string[][])  [unwired: 1 out]
            n396 = Search 1D Array(1D array=w1187, element="Seconds:since:1st Jan") -> (index of element=w1188:i32)  [unwired: 1 out]
            n397 = Increment(x=w1188) -> (x+1=w1186:i32)
            n398 = Index Array(array=w1189, index (col)=w1188) -> (element=w1190:string[])  [unwired: 1 in]
            n399 = Array Subset(array=w1189, index (col)=w1186) -> (w1199:string[][])  [unwired: 3 in]
            n400 = call "String_2_Number_array.vi"("Input String"=w1190) -> ("Values"=w1200:dbl[])
            n401 = Array Subset(array=w1187, index=w1186) -> (w1198:string[])  [unwired: 1 in]
          }
          frame #1 {
            n402 = Decimal String To Number(string=w1230) -> (number=w1201:i32)  [unwired: 3 out]
            n403 = Format Into String(format string="FF:%d:Bkgnd c^2", w1201) -> (resulting string=w1207:string)  [unwired: 2 in, 1 out]
            n404 = Search 1D Array(1D array=w1206, element=w1207) -> (index of element=w1203:i32)  [unwired: 1 in]
            n405 = Threshold 1D Array(2:w1204, 3:w1227) -> (0:w1212:dbl)  [unwired: 1 out]
            n406 = case shown="-1" w1203 {
              tunnel: w1213 -> [_ w1245]
              tunnel: w1212 -> [_ w1241]
              tunnel: [0.22 w1242] -> w1208
              tunnel: w1203 -> [_ w1240]
              tunnel: [w1238 w1240] -> w1202
              tunnel: w1201 -> [w1238 _]
              frame -1 {
              }
              frame 1, Default {
                n407 = Index Array(array=w1245, index (col)=w1240) -> (element=w1244:string[])  [unwired: 1 in]
                n408 = call "String_2_Number_array.vi"("Input String"=w1244) -> ("Values"=w1243:dbl[])
                n409 = Interpolate 1D Array(1:w1241, 2:w1243) -> (0:w1242:dbl)
              }
            }
            n410 = Decrement(x=w1202) -> (x-1=w1229:i32)
            n411 = Index Array(array=w1213, index (col)=w1229) -> (element=w1228:string[])  [unwired: 1 in]
            n412 = for {
              tunnel: w1228 -> [w1237] mode=indexing
              tunnel: [w1236] -> w1226 mode=indexing
              n413 = call "String_2_Number.vi"("Value"=w1237) -> ("Numeric"=w1236:dbl)
            }
            n414 = Interpolate 1D Array(1:w1212, 2:w1226) -> (0:w1218:dbl)
            n415 = Build Array(w1218) -> (w1222:dbl[])
            n416 = Format Into String(format string="Bkgnd Index %.2f; ", initial string=w1215, w1212) -> (resulting string=w1214:string)  [unwired: 1 in, 1 out]
            n417 = call "2nd_order_Poly_convert.vi"("Calib constants"=w1219, "Voltage"=w1222) -> ("Eng Values"=w1221:dbl[])  [unwired: 4 out]
            n418 = Index Array(array=w1221, index=0) -> (element=w1217:dbl)
            n419 = Replace Array Subset(array=w1219, new element=w1217, index=3) -> (w1210:dbl[])
            n420 = Replace Array Subset(array=w1210, new element=w1208, index=4) -> (w1209:dbl[])
          }
        }
      }
      frame "Add FFID Bkgnd Values" {
        n421 = global read "Plug_in_data_global.vi" "FFID Bkgnd Values"() -> (w1252:dbl[])
        n422 = global read "Dynamic_call_global.ph.vi" "Per Block Plug Ins"() -> (w1251:string[])
        n423 = Array Size(array=w1252) -> (size(s)=w1259:i32)
        n424 = Search 1D Array(1D array=w1251, element="Puff_Dose.vi") -> (index of element=w1249:i32)  [unwired: 1 in]
        n425 = Greater Than 0?(x=w1259) -> (x > 0?=w1247:bool)
        n426 = Less Than 0?(x=w1249) -> (x < 0?=w1248:bool)
        n427 = And(x=w1247, y=w1248) -> (x .and. y?=w1246:bool)
        n428 = case shown="True" w1246 {
          tunnel: w1258 -> [w1267 w1282]
          tunnel: [w1267 w1281] -> w1257
          tunnel: w1252 -> [_ w1276]
          tunnel: w1256 -> [w1266 w1277]
          tunnel: [w1266 w1275] -> w1255
          frame False {
          }
          frame True {
            # "20 blocks of 3 sec bkgnd"
            n429 = Index Array(array=w1276, index=0) -> (element=w1274:dbl)
            n430 = Not A Number/Path/Refnum?(number/path/refnum=w1274) -> (NaN/Path/Refnum?=w1273:bool)
            n431 = case shown="False" w1273 {
              tunnel: w1282 -> [w1285 w1287]
              tunnel: [w1284 w1287] -> w1281
              tunnel: w1274 -> [w1283 _]
              frame False {
                n432 = Replace Array Subset(array=w1285, new element=w1283, index=3) -> (w1284:dbl[])
              }
              frame True {
              }
            }
            n433 = Index Array(array=w1276, index=1) -> (element=w1271:dbl)
            n434 = Index Array(array=w1276, index=2) -> (element=w1269:dbl)
            n435 = Array Subset(array=w1276, index=3) -> (w1278:dbl[])  [unwired: 1 in]
            n436 = global write "Plug_in_data_global.vi" "FFID Bkgnd Values"(w1278) -> ()
            n437 = Format Into String(format string="%.0f blocks of %.0f Sec Bkgnd; ", initial string=w1277, w1271, w1269) -> (resulting string=w1275:string)  [unwired: 1 in, 1 out]
          }
        }
      }
      frame "Add Drift Info" {
        w1289 = T9 18 items=["0 Coeff A", "1 Coeff B", "2 Coeff C", "3 FFID Bkgnd", "4 FFID Bkgnd Variance", "5 FFID Bkgnd Volts", "6 FFID Bkgnd Time", "7 GMU Source ppm/%density", "8 Orig Bkgnd Time", "9 Orig Bknd volts", "10 Orig bkgnd Variance", "11 Intermittency Theshold", "12 Intermittency", "13 Head Temp", "14 Exhaust Temp", "15", "16", "17", "18 Calibration Drift %", "19 Calibration Interval Minutes"] ("FFID")
        n438 = call "Get_Characters_from_string.vi"("Show Dialog?"=FALSE, "Input string"=w1302, "Variable name"=w1288) -> ("Status"=w1308:enum16{"Char in string", "Char not in string"}, "Value"=w1309:string)
        n439 = Empty String/Path?(string/path=w1298) -> (empty?=w1297:bool)
        n440 = case shown="\"Char in string\"" w1308 {
          tunnel: [w1350 nan ("Value")] -> w1301
          tunnel: w1309 -> [w1346 _]
          frame "Char in string" {
            n441 = Match Pattern(string=w1346, regular expression="Drift_Place_Holder") -> (offset past match=w1348:i32)  [unwired: 4 out]
            n442 = Greater Than 0?(x=w1348) -> (x > 0?=w1347:bool)
            n443 = case shown="False" w1347 {
              tunnel: [w1351 nan ("Value")] -> w1350
              tunnel: w1346 -> [w1352 _]
              frame False {
                n444 = call "String_2_Number.vi"("Value"=w1352) -> ("Numeric"=w1351:dbl)
              }
              frame True {
              }
            }
          }
          frame "Char not in string" {
          }
        }
        n445 = case shown="False" w1297 {
          tunnel: w1298 -> [w1338 _]
          tunnel: w1292 -> [w1341 w1343]
          tunnel: [w1340 w1343] -> w1291
          frame False {
            n446 = Build Array("Correction:Info" ("string")) -> (w1339:string[])
            n447 = Build Array(w1338) -> (w1337:string[])
            n448 = call "Update Metadata channels.vi"("Metadata Values"=w1337, "Metadata Names"=w1339, "Analysis info Cluster in"=w1341) -> ("Analysis info Cluster out"=w1340:T1)
          }
          frame True {
          }
        }
        n449 = call "Get_value_from_string.vi"("Show Dialog?"=FALSE, "Input string"=w1302, "Variable name"="Minutes Until Next calibration") -> ("Status"=w1305:enum16{"Char in string", "Char not in string"}, "Value"=w1306:dbl)
        n450 = Array Size(array=w1310) -> (size(s)=w1311:i32)
        n451 = case shown="\"Char in string\"" w1305 {
          tunnel: [w1344 nan ("Value")] -> w1300
          tunnel: w1306 -> [w1344 _]
          frame "Char in string" {
          }
          frame "Char not in string" {
          }
        }
        n452 = Subtract(x=w1289, y=w1311) -> (x-y=w1312:i32)
        n453 = Initialize Array(0.0 ("Element Data"), w1312) -> (w1314:dbl[])
        n454 = Build Array (concatenate)(w1310, w1314, w1301, w1300) -> (w1296:dbl[])
        n455 = case shown="Default" w1290 {
          tunnel: ["Add FFID Metadata" "Add Zero offset info"] -> w1316
          frame "Fast FID" {
          }
          frame Default {
          }
        }
        n456 = case shown="False" w1294 {
          tunnel: w1295 -> [w1323 _]
          tunnel: w1293 -> [w1322 _]
          frame False {
            n457 = case shown="\"Psi_eff = f(Umagn.)\", \"Psi_eff, k = f(Umagn.)\"" w1322 {
              selector: w1322 -> [_ w1330 _]
              tunnel: w1323 -> [_ w1333 _]
              frame "Triangle mesh", "Polynomial surface" {
              }
              frame "Psi_eff = f(Umagn.)", "Psi_eff, k = f(Umagn.)" {
                n458 = Strip Path(path=w1333) -> (stripped path=w1328:path)  [unwired: 1 out]
                n459 = Build Path(base path=w1328, name or relative path="XW_Map.txt") -> (appended path=w1331:path)
                n460 = Build Path(base path=w1328, name or relative path="XW_Map_CALPTS.txt") -> (appended path=w1327:path)
                n461 = call "Does_file_exist_(simple).vi"("Pathname"=w1331) -> ("exists?"=w1326:bool)
                n462 = call "Does_file_exist_(simple).vi"("Pathname"=w1327) -> ("exists?"=w1325:bool)
                n463 = And(x=w1326, y=w1325) -> (x .and. y?=w1324:bool)
                n464 = case shown="True" w1324 {
                  tunnel: w1330 -> [_ w1335]
                  frame False {
                    n465 = global write "XW_Map_Global.vi" "Map method"(Map_method."Const. Psi_eff (std.)" ("Map method")) -> ()
                  }
                  frame True {
                    n466 = call "XW_Higher_order_Psi_k_PreProc_PN.vi"("Map method"=w1335) -> ()  [unwired: 1 in, 1 out]
                  }
                }
              }
              frame "Const. Psi_eff (std.)" {
                n467 = global write "XW_Map_Global.vi" "Map method"(Map_method."Const. Psi_eff (std.)" ("Map method")) -> ()
              }
            }
          }
          frame True {
          }
        }
      }
      frame "Add FFID Metadata" {
        n468 = Index Array(array=w1364, index (col)=10 ("disabled index (col)")) -> (element=w1362:dbl[])  [unwired: 1 in]
        n469 = Index Array(array=w1364, index (col)=14 ("disabled index (col)")) -> (element=w1359:dbl[])  [unwired: 1 in]
        n470 = call-poly <vilib>:"Mean.vi"("X"=w1362) -> ("mean"=w1361:dbl)  [unwired: 1 out]
        n471 = call-poly <vilib>:"Mean.vi"("X"=w1359) -> ("mean"=w1356:dbl)  [unwired: 1 out]
        n472 = Replace Array Subset(array=w1363, new element=w1361, index=14) -> (w1357:dbl[])
        n473 = Replace Array Subset(array=w1357, new element=w1356, index=15) -> (w1355:dbl[])
      }
      frame "Add Zero offset info" {
        n474 = call "Get_Calib_zero_Offset.vi"("Measurement Time"=w1375, "Calib Filename"=w1385) -> ("Voltage Offset"=w1382:dbl)
        n475 = Not A Number/Path/Refnum?(number/path/refnum=w1382) -> (NaN/Path/Refnum?=w1384:bool)
        n476 = case shown="False" w1384 {
          tunnel: w1383 -> [w1397 w1433]
          tunnel: w1378 -> [w1396 w1432]
          tunnel: w1382 -> [w1395 _]
          tunnel: [w1394 0.0 ("Time Data was Aquired")] -> w1377
          tunnel: [w1393 w1431] -> w1376
          frame False {
            n477 = case shown="\"Fast FID\"" w1397 {
              tunnel: w1396 -> [_ _ _ _ w1404 w1412 w1417 w1424 _ _ _ _]
              tunnel: w1395 -> [_ _ _ _ w1407 w1410 w1419 w1422 _ _ _ _]
              tunnel: [w1398 w1399 w1400 w1401 1.0 ("Time Data was Aquired") 1.0 ("Time Data was Aquired") 1.0 ("Time Data was Aquired") 1.0 ("Time Data was Aquired") w1426 w1427 w1428 w1429] -> w1394
              tunnel: [w1398 w1399 w1400 w1401 w1403 w1409 w1415 w1421 w1426 w1427 w1428 w1429] -> w1393
              frame "Raw voltage" {
                w1398 = 0.0 ("Time Data was Aquired")
              }
              frame "Hot wire" {
                w1399 = 0.0 ("Time Data was Aquired")
              }
              frame "Cross wire 1" {
                w1400 = 0.0 ("Time Data was Aquired")
              }
              frame "Cross wire 2" {
                w1401 = 0.0 ("Time Data was Aquired")
              }
              frame "Generic Linear", Default {
                n478 = Build Array(w1407) -> (w1406:dbl[])
                n479 = call "Linear_voltage_converter.vi"("Caib const A,B"=w1404, "Voltage array"=w1406) -> ("Converted array"=w1405:dbl[])
                n480 = Index Array(array=w1405) -> (element=w1403:dbl)  [unwired: 1 in]
              }
              frame "Generic Polynomial" {
                n481 = call "Minimum_Polynomial_Coefficents.vi"("Calib consts"=w1412, "Max Length"=6) -> ("Coefficients"=w1411:dbl[])
                n482 = call "Polynomial_convert.vi"("Calib constants"=w1411, "Voltage"=w1410) -> ("Eng Values"=w1409:dbl)  [unwired: 4 out]
              }
              frame "Fast FID" {
                n483 = Array Subset(array=w1417, length=3) -> (w1416:dbl[])  [unwired: 1 in]
                n484 = call "Polynomial_convert.vi"("Calib constants"=w1416, "Voltage"=w1419) -> ("Eng Values"=w1415:dbl)  [unwired: 4 out]
              }
              frame "Generic BackPoly" {
                n485 = Array Subset(array=w1424, length=6) -> (w1423:dbl[])  [unwired: 1 in]
                n486 = call "Polybackwards.vi"("Coefficients"=w1423, "Y input"=w1422) -> ("X output"=w1421:dbl)  [unwired: 1 out]
              }
              frame "Thermocouple" {
                w1426 = 0.0 ("Time Data was Aquired")
              }
              frame "Cold wire" {
                w1427 = 0.0 ("Time Data was Aquired")
              }
              frame "Pulsed Wire" {
                w1428 = 0.0 ("Time Data was Aquired")
              }
              frame "Microphone" {
                w1429 = 0.0 ("Time Data was Aquired")
              }
            }
          }
          frame True {
            n487 = case shown="\"Fast FID\"" w1433 {
              tunnel: w1432 -> [w1436 _]
              tunnel: [w1434 0.0 ("Time Data was Aquired")] -> w1431
              frame "Fast FID" {
                n488 = Index Array(array=w1436, index=3) -> (element=w1434:dbl)
              }
              frame "Raw voltage", Default {
              }
            }
          }
        }
        n489 = Build Array (concatenate)(w1378, w1377, w1376) -> (w1379:dbl[])
      }
    }
  }
  "Calib Coeff" <- w27
  "Analysis Info cluster  Out" <- w11
